vi "Text control 2 v4.3_pump-specific.vi"() -> ()   [LabVIEW 2016]
panel:
  in  "Tab Control":enum32{"Main", "Other parameters"}(tab)
  out "Line running":i32
  out "Total lines":i32
  out "Path":path=path "C:/users/rlp38/09Apr2009LTtesting/test2.txt"
  out "I vs Vg":cluster{"Y data in":dbl[], "X data in":dbl[]}[](graph)
  out "Is":dbl format="%.2e"
  out "Id":dbl format="%.2e"
  out "Ig":dbl format="%.2e"
  out "Id max vs time":cluster{"Y data in":dbl[], "X data in":dbl[]}[](graph)
  out "Id min vs time":cluster{"Y data in":dbl[], "X data in":dbl[]}[](graph)
  out "I vs Vd":cluster{"Y data in":dbl[], "X data in":dbl[]}[](graph)
  in  "Program":string="#pulsedstressV d 0.03 20 0 0.5 0.0827 5\n#\n#itime s\n#gaterangemode l\n#drainrangemode l\n#serial /1Q #query pump\n#wait 1000 #wait 1 second\n#serial /1ZR #initialize pump\n#serial /1Q #query pump\n#wait 20000 #wait 20 seconds\n#serial /1N0R #set step resolution: 0.01 mm\n#serial /1Q #query pump\n#wait 1000 #wait 1 second\n#serial /1V300R #choose speed: 300 steps/s\n#serial /1Q #query pump\n#wait 1000 #wait 1 second\n#serial /1O3R #go to port 3, counterclockwise rotation\n#serial /1Q #query pump\n#wait 1000 #wait 1 second\n#serial /1A2400R #go to absolute position 2400\n#serial /1Q #query pump\n#wait 1000 #wait 1 second\n#serial /1Q #query pump\n#serial /1? #report absolute plunger position\n#serial /1V80R #set speed to 80 steps/s\n#serial /1Q #query pump\n#serial /1O5 #switch to port 5, counterclockwise rotation\n#serial /1Q #query pump\n#wait 200 #wait 200 milliseconds\n#serial /1A0R #go to absolute position 0 (= empty syringe)\n#serial /1Q #query pump\n#serial /1? #report absolute plunger position\n#pulsed on 0.05 0 0.02\n#transfer d 1 -1 -0.1 -1 -1 0\n#wait-min 1\n#transfer d 1 -1 -0.1 -1 -1 0\n#output d 0 -1 -0.5 0 -1 -0.1\n#transfer d -10 40 1 5 40 35\n#transfer d -10 40 1 5 40 35\n#output d 0 40 20 0 40 1\n#\n#\n#sample 1 0.008 221 6 0.003\n#samplei 400e-6 200 6 0.002 0.1\n#vsu2pulse -10 4\n#\n#stressV 0.016 0.03 2e-4 0.1e-3 11\n#stressI 220e-7 0.08 15\n#transfer s -1 1 0.5 -0.005 0.005 0.005\n#output s 0 0 0 -0.008 0.008 0.002"
  out "Command running:":string="#output s 0 0 0 -0.008 0.008 0.002"
  out "Serial port data":string
  out "Elapsed Time":dbl caption="Elapsed Time (s)"
  in  "Units":u16(ring) items=["Seconds", "Minutes", "Hours"]
  in  "Time Offset":dbl caption="Set Start Time (s)"
  in  "Reset":bool
  in  "Auto Reset":bool
  in  "integration time":u32(slide) max=2 step=1 scale=0.0..2.0
  in  "Interrupt run":bool
  out "Absolute plunger position vs time":cluster{"Y data in":dbl[], "X data in":dbl[]}[](graph)
  out "Valve position vs time":cluster{"Y data in":dbl[], "X data in":dbl[]}[](graph)
  in  "Gate Range\nmode":u16(ring) items=["Auto", "Limited", "Fixed"]
  in  "Gate Range":u8(slide)=6 max=11 scale=0.0..11.0
  in  "Source/Drain\nRange mode":u16(ring) items=["Auto", "Limited", "Fixed"]
  in  "Source/Drain Range":u8(slide)=6 max=11 scale=0.0..11.0
  in  "Panel Controls":T1={"Emergency Stop"=refnum, "TransGraph Max"=1e-05, "Text/Graph (text=false)"=TRUE} {"TransGraph Max" format="%.2e"}
  in  "Panel Controls 2":T2={"Emergency Stop"=refnum, "TransGraph Max"=1e-05, "Text/Graph (text=false)"=TRUE, "TransGraph Min"=1e-11} {"TransGraph Min" format="%.2e"; "TransGraph Max" format="%.2e"}
  in  "SMU4":cluster{"on/off":bool, "Voltage":dbl} {"Voltage" min=-100.0 max=100.0 format="%.2f"}
  in  "Full Reset":bool
  in  "Standby":T3
  out "error out":errorcluster
  in  "Delay before read (ms)":u32=1000
  in  "byte count":u32=64
  in  "Serial End Mode for Reads":u16(ring)=2 items=["None", "LastBit", "TermChar"]
  in  "Timeout (ms)":u32=10000
  in  "Enable Termination\nChar (T)":bool=TRUE
  in  "Termination char\n(0xA = '\\n' = LF)\n(0xD = '\\r' = CR)":u8=13 format="%.0x"
  in  "flow control":u16(ring) items=["None"=0, "XON/XOFF"=1, "RTS/CTS"=2, "DTR/DSR"=4]
  in  "stop bits":u16(ring)=10 items=["1.0"=10, "1.5"=15, "2.0"=20]
  in  "parity":u16(ring) items=["None", "Odd", "Even", "Mark", "Space"]
  in  "data bits":u16=8 min=5 max=8 step=1
  in  "VISA resource name":refnum<visa-resource-name>="COM6"
  in  "baud rate":u32=9600
  in  "Drain: Compliance":dbl=0.001 format="%.8f"
  in  "Gate: Compliance":dbl=0.001 format="%.8f"
  in  "hold time /s":dbl format="%.2f"
  in  "delay time /s":dbl format="%.2f"
  in  "Integration time (short)":dbl=0.0019 min=8e-05 max=0.0019 step=8e-05 format="%^.0e"
  in  "Integration time (long)":dbl=0.32 min=0.04 max=2.0 step=0.02 format="%.2f"
  in  "Step delay /s":dbl format="%.2f"
  in  "Prefix (transfer)":string="_step_1_air_"
  in  "Suffix (transfer)":string="_Vg=0_T_1.txt"
  in  "Prefix (time data)":string="_buffer_Idmax_Idmin_vs_time_Vg=-1.0V_Vd=-1.0V"
  in  "Suffix (time data)":string=".txt"
  in  "Prefix (output)":string="_step_1_air_"
  in  "Suffix (output)":string="_Vg=0_O_1.txt"
  in  "Gate":T4={"Gate Start"=0.0, "Gate Stop"=2.0, "Gate Step (linear only)"=1.0, "Gate Compliance"=0.0001, "Gate PComp"=0.0, "Range mode"=0, "Range"=6} {"Range" max=11 scale=0.0..11.0; "Range mode" items=["Auto", "Limited", "Fixed"]; "Gate PComp" format="%^.2e"; "Gate Compliance" format="%^.2e"; "Gate Step (linear only)" format="%^.4e"; "Gate Stop" format="%^.4e"; "Gate Start" format="%^.4e"}
  in  "Drain 2":T5={"Drain Start"=0.0, "Drain Stop"=2.0, "Drain Compliance"=0.0001, "Drain Step"=1.0, "Drain PComp"=0.0, "Range mode"=0, "Range"=6} {"Range" max=11 scale=0.0..11.0; "Range mode" items=["Auto", "Limited", "Fixed"]; "Drain PComp" format="%^.2e"; "Drain Step" format="%^.4e"; "Drain Compliance" format="%^.2e"; "Drain Stop" format="%^.4e"; "Drain Start" format="%^.4e"}
  in  "Timings 2":T6={"integration time"=0, "Short/Long integration time"=0.00064, "hold time (sec)"=0.0, "delay time (sec)"=0.0, "Step Time (0 disables)"=0.0, "sweep method"=0, "Pulse period"=0.005, "Base voltage"=0.0, "Pulse width"=0.0005} {"Pulse width" min=0.0005 max=0.1 step=0.0001 format="%.4f"; "Base voltage" format="%^.4e"; "Pulse period" min=0.005 max=1.0 step=0.0001 format="%.4f"; "sweep method" items=["Continuous", "Pulsed"]; "Step Time (0 disables)" format="%.2f"; "delay time (sec)" format="%.4f"; "hold time (sec)" format="%.4f"; "Short/Long integration time" format="%^.0e"; "integration time" scale=0.0..2.0}
  # "Syntax:\nitime [s|m|l]\ngaterangemode [a|l|f]\ndrainrangemode [a|l|f]\npulsed [on|off] PulsePeriod(sec) PulseBaseVoltage PulseONWidth(sec)\nstandby [on l off]\nwait NumMilliseconds\nwait-min NumMinutes\n# texthere = comment\ntransfer [s|d] VgStart VgStop VgStep VdStart VdStop VdStep\noutput [s|d] VgStart VgStop VgStep VdStart VdStop VdStep\nsample Vg Vd NumSamples Time(s) SampleInterval(s)\nsamplei Idg NumSamples Time(s) SampleInterval(s) VDGcompliance\n100 samples is approximately 13 seconds with medium integration\n# if in doubt use SampleInterval(s) = 0.004\nstressV VG VD IGcompliance IDcompliance Duration(sec)\nstressI IDG VDGcompliance Duration(sec)\nvsu2pulse Bias Duration(s)\npulsedstressV [s|d] VEstop VgON VgOFF Period(s) PulseONwidth(s) Vd\nsample-fpp Vg Vd NumSamples Time\nresample-fpp Vg Vd\ntransfer-fpp [s|d] VgStart VgStop VgStep VdStart VdStop VdStep\noutput-fpp [s|d] VgStart VgStop VgStep VdStart VdStop VdStep\nserial SerialPortCommand\npump SerialPortCommand for the OEM pump\nSPM OEM Pump Syntax (<x>: pump number, use 1 if only one pump):\nif the command syntax contains [R], then append the letter R to the command\n/<x>Q: query (a query command should follow each command)\n/<x>Z[R] or /<x>Y[R]: initialize pump\n/<x>N<n>[R] (<n>=0,1): <0> (<1>) microstep 0.01 mm (0.00125 mm) resolution\n/<x>I<n> (<n>=0-6): turn to port number n (clockwise)\n/<x>O<n> (<n>=0-6): turn to port number n (counterclockwise)\n/<x>X: Re-execute last command string\n/<x>G<n>[R] (<n>=0-60000): repeat command sequence (default: 0, 0=loop forever)\n/<x>g: Mark the start of a repeat sequence (max = 10)\n/<x>M<n>[R] (<n>=0-86400000): delay command execution by n milliseconds\n/<x>H: Halt; Pause the sequence after finishing the current move\n/<x>T: Hardstop; Interrupt the current move and suppress it from the sequence\n/<x>A<n>[R] (<n>=0-3000 with N=0, 0-24000 with N=1): absolute position\n/<x>P<n>[R] (<n>=0-3000 with N=0, 0-24000 with N=1): relative pickup\n/<x>D<n>[R] (<n>=0-3000 with N=0, 0-24000 with N=1): relative dispense\n/<x>V<n>[R] (<n>=5-1600 default: 150): set peak speed (pulses/sec)\n/<x>S<n>[R] (<n>=10-40 default: 22): set speed (NOT in pulses/sec, look in manual)\nNOTE: When controlled with absolute position, one does not need to pay special attention to the syringe that is mounted on the pump.\nWithdraw from lower stage (ports 1, 3, 5), dispense from higher stage (ports 2, 4, 6)."
  # "Time"
  # "1\n2\n3\n4\n5\n6\n7\n8\n9\n10\n11\n12\n13\n14\n15\n16\n17\n18\n19\n20"
  # "Serial port settings"
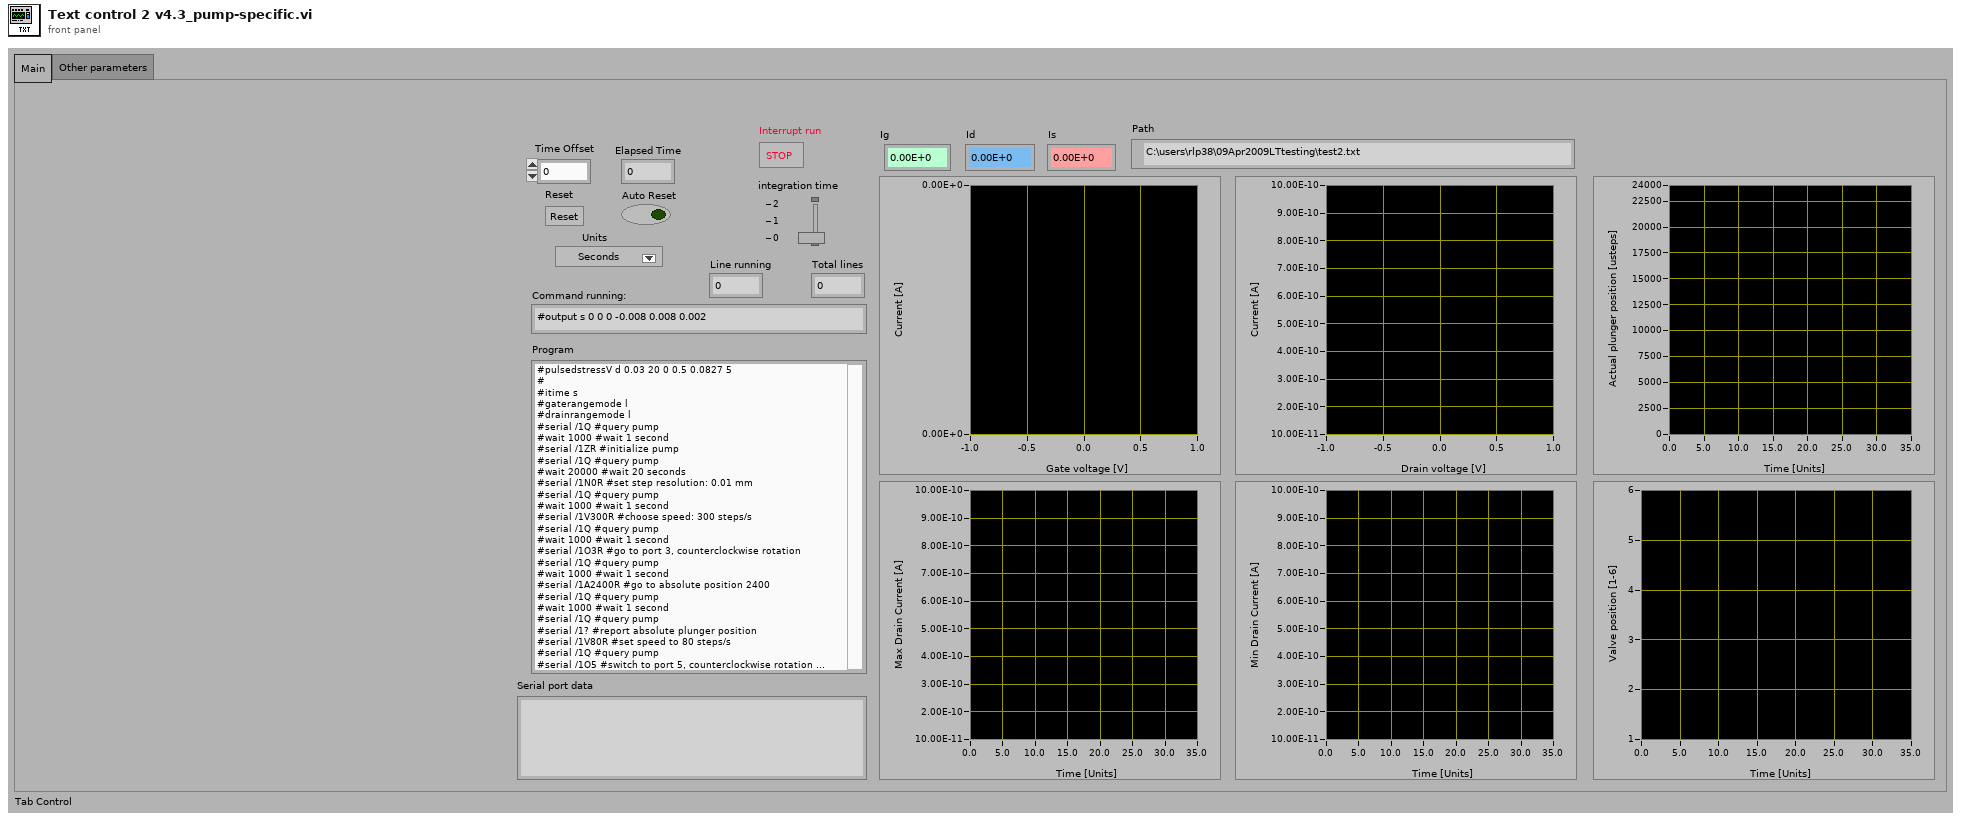
[diagram p1: front panel]
types:
  T1 = cluster{"Emergency Stop":refnum<vi>, "TransGraph Max":dbl, "Text/Graph (text=false)":bool}
  T2 = cluster{"Emergency Stop":refnum<vi>, "TransGraph Max":dbl, "Text/Graph (text=false)":bool, "TransGraph Min":dbl}
  T3 = cluster{"Gate Standby":bool, "Drain Standby":bool}
  T4 = cluster{"Gate Start":dbl, "Gate Stop":dbl, "Gate Step (linear only)":dbl, "Gate Compliance":dbl, "Gate PComp":dbl, "Range mode":u16, "Range":u8}
  T5 = cluster{"Drain Start":dbl, "Drain Stop":dbl, "Drain Compliance":dbl, "Drain Step":dbl, "Drain PComp":dbl, "Range mode":u16, "Range":u8}
  T6 = cluster{"integration time":u32, "Short/Long integration time":dbl, "hold time (sec)":dbl, "delay time (sec)":dbl, "Step Time (0 disables)":dbl, "sweep method":u16, "Pulse period":dbl, "Base voltage":dbl, "Pulse width":dbl}
  T7 = enum16{"open", "replace", "create", "open or create", "replace or create", "replace or create with confirmation"}
  T8 = cluster{"V2 Start":dbl, "V2 Step":dbl, "Number of points":i32}
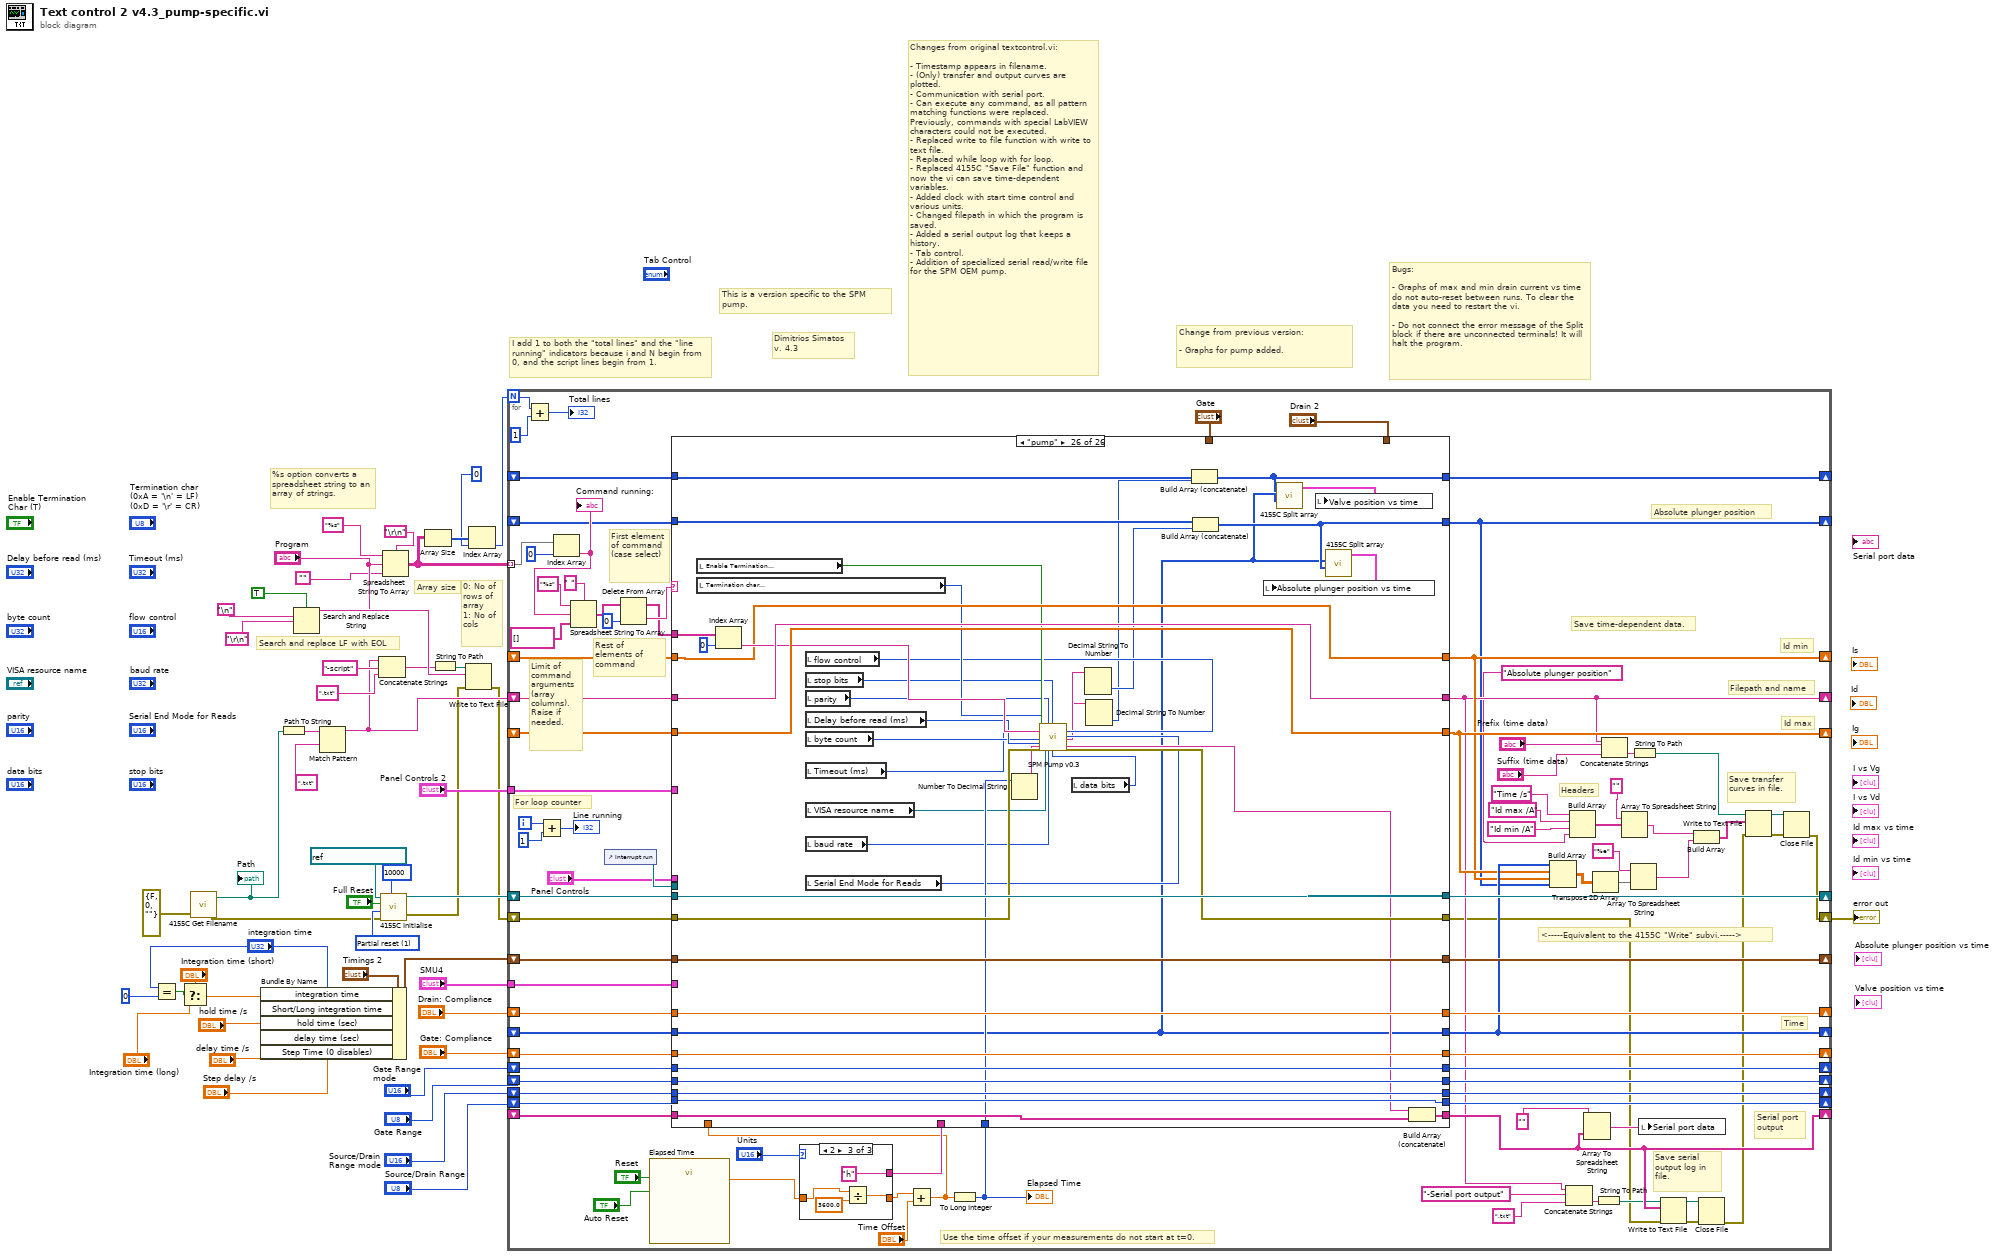
[diagram p0: block diagram]
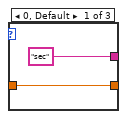
[diagram p2: hidden frame]
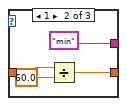
[diagram p3: hidden frame]
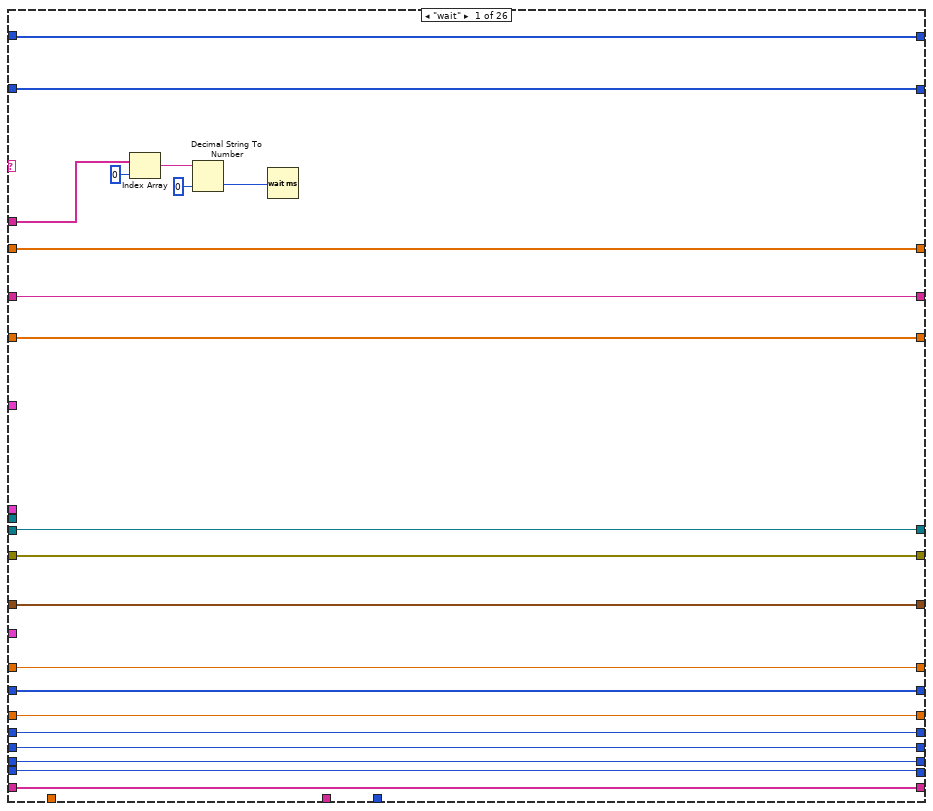
[diagram p4: hidden frame]
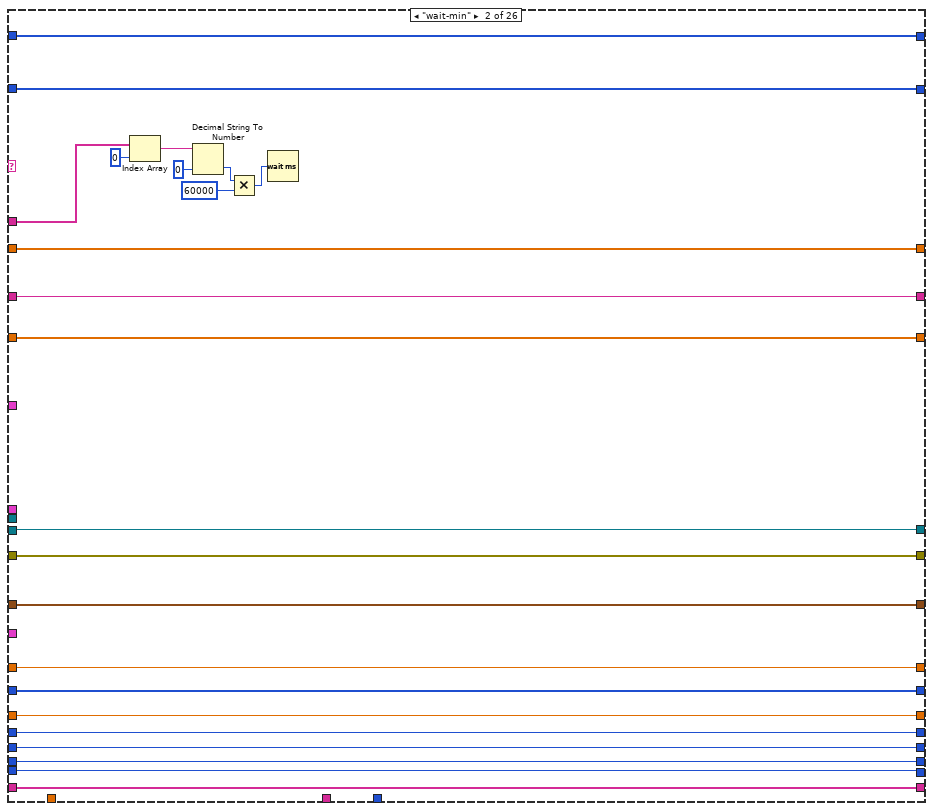
[diagram p5: hidden frame]
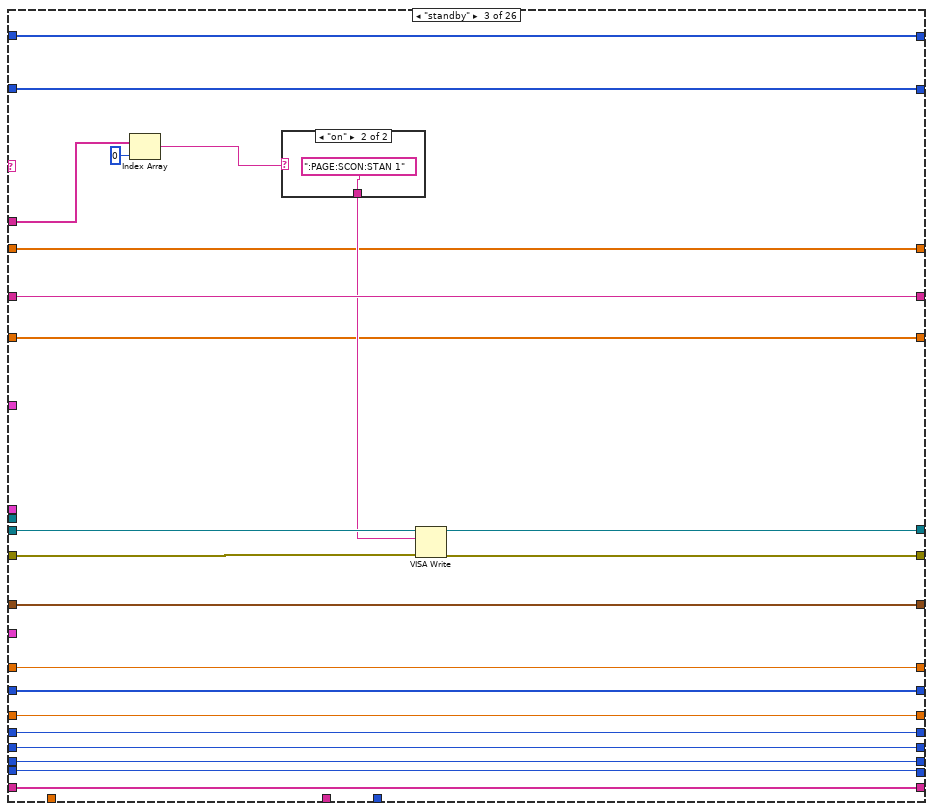
[diagram p6: hidden frame]
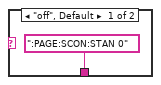
[diagram p7: hidden frame]
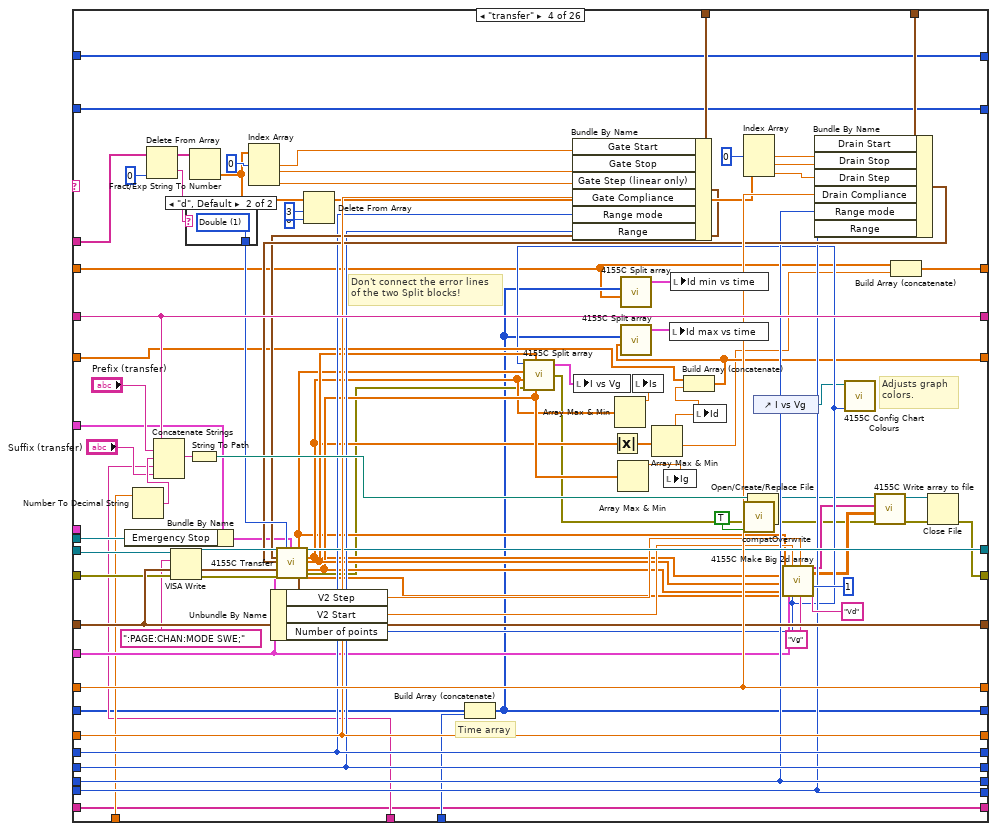
[diagram p8: hidden frame]
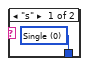
[diagram p9: hidden frame]
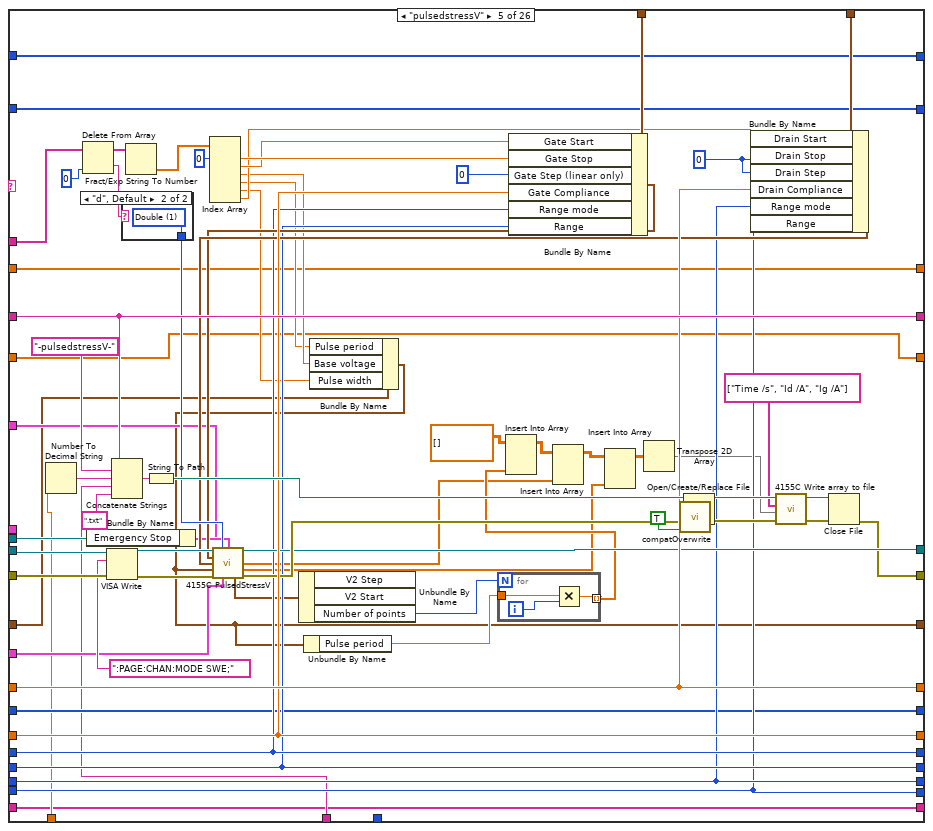
[diagram p10: hidden frame]
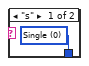
[diagram p11: hidden frame]
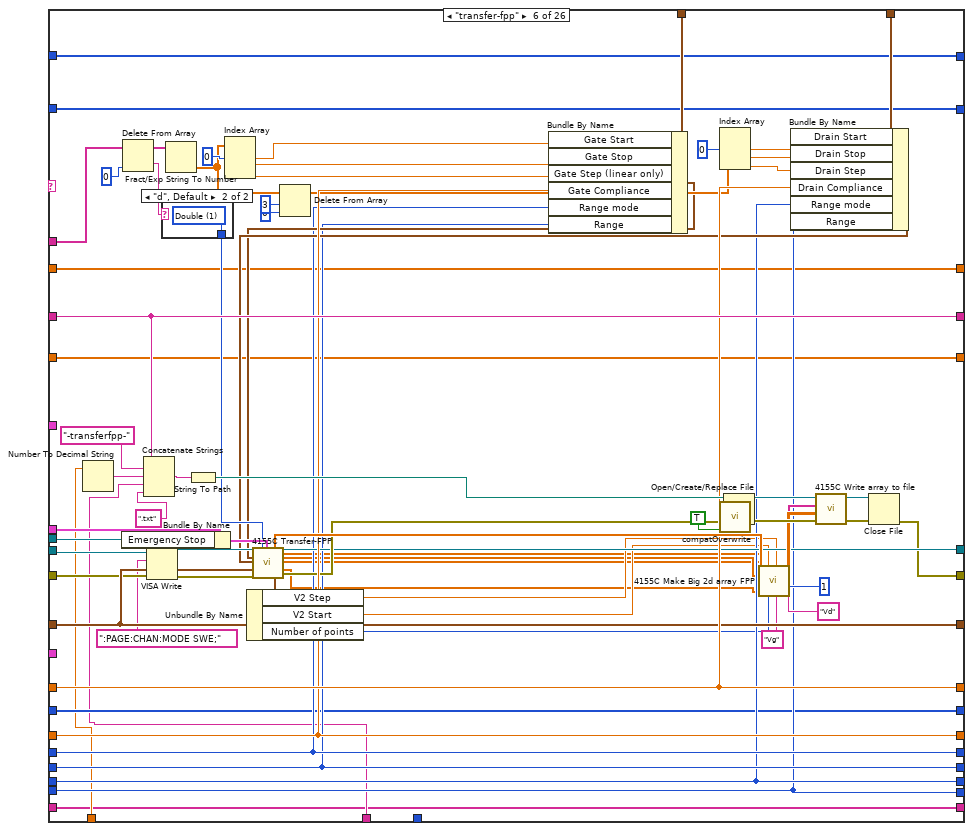
[diagram p12: hidden frame]
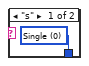
[diagram p13: hidden frame]
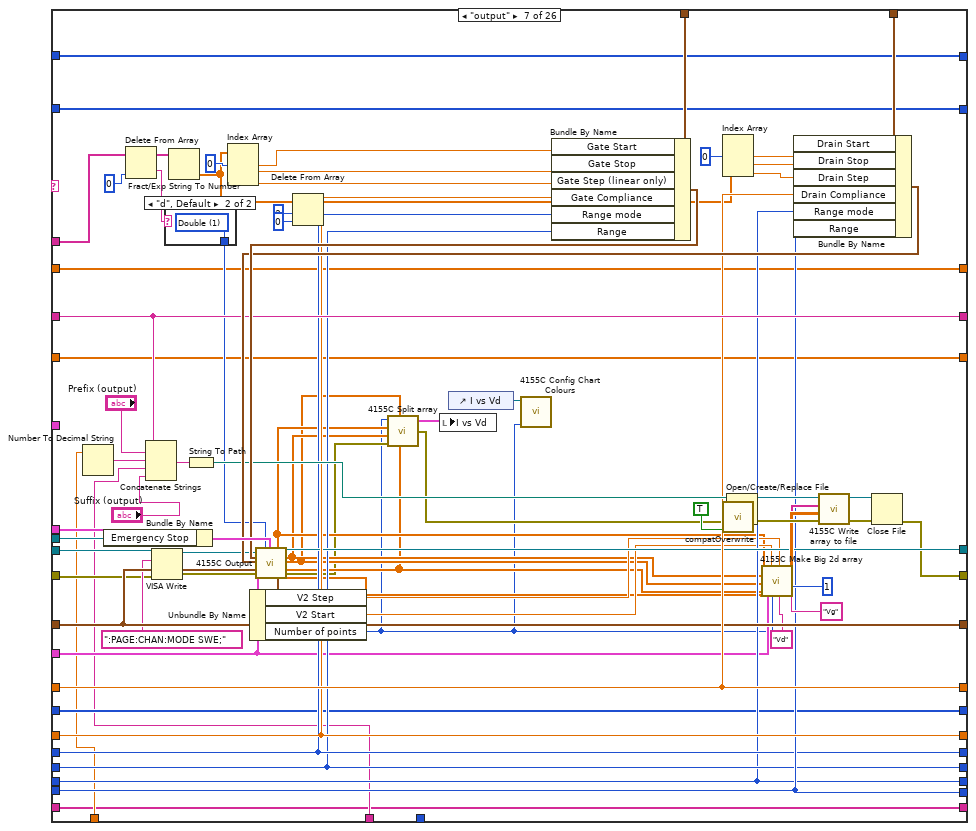
[diagram p14: hidden frame]
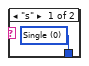
[diagram p15: hidden frame]
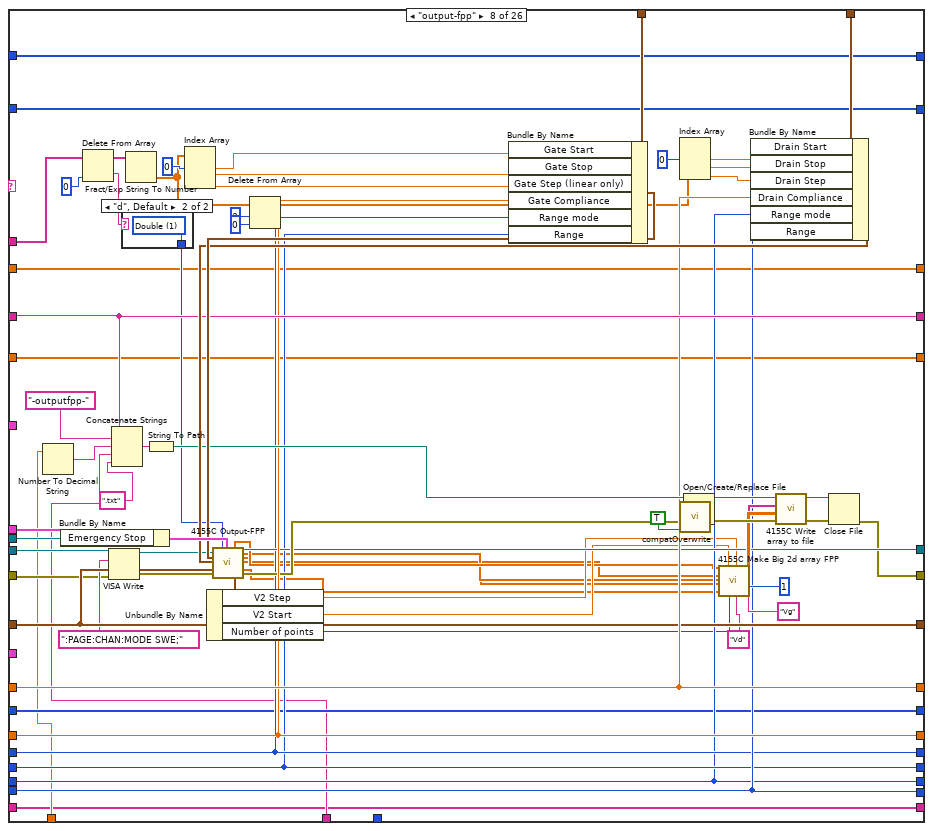
[diagram p16: hidden frame]
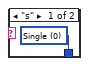
[diagram p17: hidden frame]
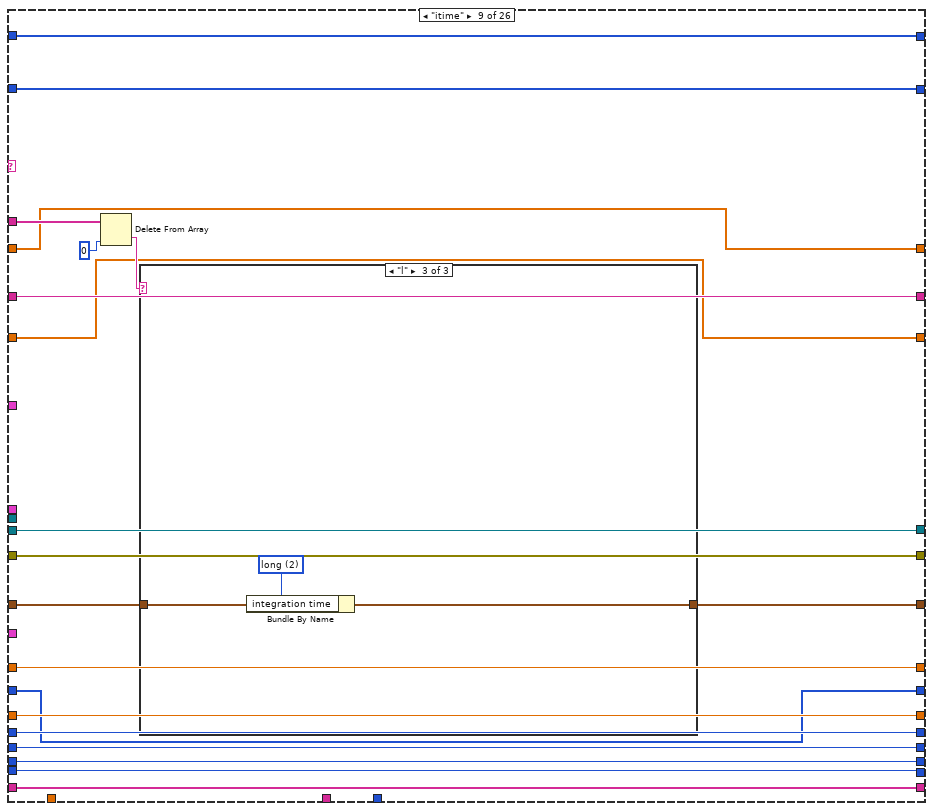
[diagram p18: hidden frame]
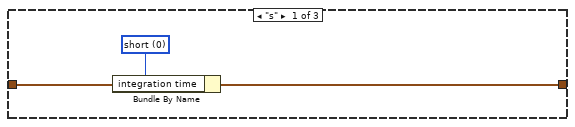
[diagram p19: hidden frame]
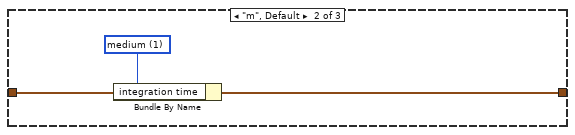
[diagram p20: hidden frame]
diagram:
  w40 = u16 1 items=["Reset All", "Partial reset"] ("Type of reset")
  # "This is a version specific to the SPM pump."
  # "I add 1 to both the \"total lines\" and the \"line running\" indicators because i and N begin from 0, and the script lines begin from 1."
  # "Bugs:\n\n- Graphs of max and min drain current vs time do not auto-reset between runs. To clear the data you need to restart the vi.\n\n- Do not connect the error message of the Split block if there are unconnected terminals! It will halt the program."
  # "Array size"
  # "%s option converts a spreadsheet string to an array of strings."
  # "0: No of rows of array\n1: No of cols"
  # "Change from previous version:\n\n- Graphs for pump added."
  # "Dimitrios Simatos\nv. 4.3"
  # "Changes from original textcontrol.vi:\n\n- Timestamp appears in filename.\n- (Only) transfer and output curves are plotted.\n- Communication with serial port.\n- Can execute any command, as all pattern matching functions were replaced. Previously, commands with special LabVIEW characters could not be executed.\n- Replaced write to file function with write to text file.\n- Replaced while loop with for loop.\n- Replaced 4155C \"Save File\" function and now the vi can save time-dependent variables.\n- Added clock with start time control and various units.\n- Changed filepath in which the program is saved.\n- Added a serial output log that keeps a history.\n- Tab control.\n- Addition of specialized serial read/write file for the SPM OEM pump."
  # "Search and replace LF with EOL"
  n1 = Equal?(x="integration time", y=u32 0) -> (x = y?=w44:bool)
  n2 = Select(t="Integration time (short)", s=w44, f="Integration time (long)") -> (s? t:f=w48:dbl)
  n3 = call "4155C Get Filename.vi"("error in (no error)"=errorcluster {"status"=FALSE, "code"=0, "source"=""}) -> ("error out"=w35:errorcluster, "path"=w10:path)  [unwired: 2 in, 1 out]
  "Path" <- w10
  n4 = Bundle By Name(cluster="Timings 2", "integration time"="integration time", "Short/Long integration time"=w48, "hold time (sec)"="hold time /s", "delay time (sec)"="delay time /s", "Step Time (0 disables)"="Step delay /s") -> (w33:T6)
  n5 = Path To String(path=w10) -> (string=w11:string)
  n6 = Search and Replace String(replace all?=TRUE ("replace all? (F)"), input string="Program", search string="\n", replace string="\r\n") -> (result string=w23:string)  [unwired: 4 in, 3 out]
  n7 = Match Pattern(string=w11, regular expression=".txt") -> (before substring=w5:string)  [unwired: 1 in, 3 out]
  n8 = Concatenate Strings(w5, "-script" ("Prefix"), ".txt" ("regular expression")) -> (w4:string)
  n9 = call "4155C Initialise.vi"("VISA resource name in"=refnum<visa-resource-name> "GPIB0::14::INSTR", "Reset"="Full Reset", "Type of reset"=w40, "error in (no error)"=w35, "VISA Timeout Value"=u32 10000) -> ("VISA Resource Name out"=w34:refnum<visa-resource-name>, "error out"=w2:errorcluster)
  n10 = Spreadsheet String To Array(delimiter (Tab)="\r\n", format string="%s", spreadsheet string="Program", array type (2D Dbl)="") -> (array=w14:string[][])
  n11 = Array Size(array=w14) -> (size(s)=w18:i32[])
  n12 = String To Path(string=w4) -> (path=w3:path)
  n13 = Write to Text File(file (use dialog)=w3, text=w23, error in=w2) -> (error out=w1:errorcluster)  [unwired: 1 in, 2 out]
  n14 = Index Array(array=w18, index=0) -> (element=w16:i32)
  n15 = for {
    N: w16 -> [w73]
    tunnel: "SMU4" -> [w118]
    shift-left: "Source/Drain Range" -> [w123]
    shift-right: [w119] -> _
    shift-left: "Source/Drain\nRange mode" -> [w124]
    shift-right: [w120] -> _
    shift-left: "Gate Range" -> [w125]
    shift-right: [w121] -> _
    shift-left: "Gate Range\nmode" -> [w126]
    shift-right: [w122] -> _
    shift-left: "Gate: Compliance" -> [w135]
    shift-right: [w131] -> _
    shift-left: "Drain: Compliance" -> [w136]
    shift-right: [w132] -> _
    shift-left: w33 -> [w137]
    shift-right: [w133] -> _
    shift-left: w1 -> [w138]
    shift-right: [w81] -> w9
    shift-left: w34 -> [w139]
    shift-right: [w134] -> _
    shift-left: w5 -> [w140]
    shift-right: [w57] -> _
    tunnel: "Panel Controls 2" -> [w117]
    shift-right: [w85] -> _
    shift-left: _ -> [w116]
    shift-right: [w86] -> _
    shift-left: _ -> [w112]
    tunnel: w14 -> [w110] mode=indexing
    shift-right: [w79] -> _
    shift-left: _ -> [w80]
    shift-right: [w62] -> _
    shift-left: _ -> [w65]
    shift-right: [w53] -> _
    shift-left: _ -> [w54]
    shift-right: [w51] -> _
    shift-left: _ -> [w50]
    i -> [w68]
    # "Absolute plunger position"
    # "Serial port output"
    # "Save serial output log in file."
    # "For loop counter"
    # "<-----Equivalent to the 4155C \"Write\" subvi.----->"
    # "Headers"
    # "Save transfer curves in file."
    # "Filepath and name"
    # "Save time-dependent data."
    # "Use the time offset if your measurements do not start at t=0."
    # "Time"
    # "Rest of elements of command"
    # "Id min"
    # "Id max"
    # "Limit of command arguments (array columns). Raise if needed."
    # "First element of command\n(case select)"
    n16 = Add(x=w73, y=1) -> (x+y=→"Total lines":i32)
    n17 = Add(x=w68, y=1) -> (x+y=→"Line running":i32)
    n18 = Index Array(array=w110, index=0 ("line index")) -> (element=w105:string)
    "Command running:" <- w105
    n19 = Spreadsheet String To Array(delimiter (Tab)=" ", format string="%s", spreadsheet string=w105, array type (2D Dbl)=string[] []) -> (array=w102:string[])
    n20 = control-ref of="Interrupt run"() -> (w130:refnum<vi>)
    n21 = Delete From Array(array=w102, index=0) -> (deleted portion=w103:string, array with subset deleted=w101:string[])  [unwired: 1 in]
    n22 = call "Elapsed Time"("Reset"="Reset", "Auto Reset"="Auto Reset") -> ("Elapsed Time (s)"=w113:dbl)  [unwired: 10 in, 7 out]
    n23 = case shown="2" "Units" {
      tunnel: ["sec" "min" "h"] -> w114
      tunnel: [w141 w145 w148] -> w75
      tunnel: w113 -> [w141 w144 w149]
      frame 0, Default {
      }
      frame 1 {
        n24 = Divide(x=w144, y=60.0) -> (x/y=w145:dbl)
      }
      frame 2 {
        n25 = Divide(x=w149, y=3600.0) -> (x/y=w148:dbl)
      }
    }
    n26 = Add(x=w75, y="Time Offset") -> (x+y=w74:dbl)
    n27 = To Long Integer(number=w74) -> (32bit integer=w111:i32)
    "Elapsed Time" <- w111
    n28 = case shown="\"pump\"" w103 {
      tunnel: w101 -> [w171 w194 w216 w295 w363 w436 w515 w589 w631 w661 w692 w721 w746 w764 _ _ w880 w945 _ w1018 w1066 w1112 w1186 w1252 w1276 w1321]
      tunnel: w140 -> [w166 w190 w214 w302 w370 w444 w522 w597 w620 w650 w684 w714 w740 w757 w780 w826 w858 w927 w962 w1005 w1053 w1100 w1180 w1248 w1278 w1323]
      tunnel: w139 -> [w165 w189 w205 w273 w354 w413 w491 w565 w621 w651 w685 w715 w741 w758 w785 w828 w886 w951 w966 w1024 w1072 w1118 w1192 w1206 w1282 w1327]
      tunnel: w138 -> [w164 w188 w204 w272 w353 w412 w488 w562 w622 w652 w686 w716 w742 w759 w784 w799 w885 w950 w965 w1023 w1071 w1117 w1191 w1205 w1281 w1326]
      tunnel: w137 -> [w163 w187 w213 w298 w329 w440 w518 w593 w630 w660 w683 w713 w739 w756 w783 w823 w849 w919 w971 w998 w1046 w1093 w1179 w1247 w1283 w1328]
      tunnel: w136 -> [w162 w186 w212 w300 w368 w442 w520 w595 w629 w659 w691 w720 w745 w763 w782 w808 w884 w949 w974 w1022 w1070 w1116 w1190 w1256 w1284 w1329]
      tunnel: w135 -> [w161 w185 w211 w299 w367 w441 w519 w594 w628 w658 w690 w719 w744 w762 w781 w809 w859 w928 w973 w1006 w1054 w1101 w1181 w1249 w1286 w1330]
      tunnel: [w165 w189 w203 w297 w365 w438 w517 w591 w621 w651 w685 w715 w741 w758 w785 w828 w850 w901 w964 w999 w1047 w1094 w1132 w1208 w1282 w1327] -> w134
      tunnel: [w164 w188 w202 w296 w364 w437 w516 w590 w622 w652 w686 w716 w742 w759 w784 w798 w860 w902 w963 w1007 w1055 w1102 w1131 w1207 w1280 w1325] -> w56
      tunnel: [w163 w187 w213 w298 w325 w440 w518 w593 w623 w653 w683 w713 w739 w756 w783 w823 w849 w919 w971 w998 w1046 w1093 w1179 w1247 w1283 w1328] -> w133
      tunnel: [w162 w186 w212 w300 w368 w442 w520 w595 w629 w659 w691 w720 w745 w763 w782 w808 w884 w949 w974 w1022 w1070 w1116 w1190 w1256 w1284 w1329] -> w132
      tunnel: [w161 w185 w211 w299 w367 w441 w519 w594 w628 w658 w690 w719 w744 w762 w781 w809 w859 w928 w973 w1006 w1054 w1101 w1181 w1249 w1286 w1330] -> w131
      tunnel: [w166 w190 w214 w302 w370 w444 w522 w597 w620 w650 w684 w714 w740 w757 w780 w826 w858 w927 w962 w1005 w1053 w1100 w1180 w1248 w1278 w1323] -> w57
      tunnel: w130 -> [_ _ _ w305 w374 w449 w526 w601 _ _ _ _ _ _ _ _ w855 w924 _ w1004 w1052 w1099 w1152 w1224 _ _]
      tunnel: "Gate" -> [_ _ _ w282 w357 w423 w502 w576 _ _ _ _ _ _ _ _ _ _ _ _ _ _ _ _ _ _]
      tunnel: "Drain 2" -> [_ _ _ w281 w356 w422 w501 w575 _ _ _ _ _ _ _ _ _ _ _ _ _ _ _ _ _ _]
      tunnel: "Panel Controls" -> [_ _ _ _ _ w421 w500 w574 _ _ _ _ _ _ _ _ _ _ _ _ _ _ _ _ _ _]
      tunnel: w126 -> [w160 w184 w210 w266 w347 w406 w486 w560 w627 w657 _ w712 w738 w755 w779 w810 w845 w915 w967 w994 w1042 w1089 w1175 w1243 w1287 w1331]
      tunnel: w125 -> [w159 w183 w209 w265 w346 w405 w485 w559 w626 w656 w689 _ w729 w761 w778 w811 w846 w916 w968 w995 w1043 w1090 w1176 w1244 w1288 w1332]
      tunnel: w124 -> [w158 w182 w208 w264 w345 w404 w484 w558 w625 w655 w688 w718 w743 _ w777 w812 w847 w917 w969 w996 w1044 w1091 w1177 w1245 w1289 w1333]
      tunnel: w123 -> [w157 w181 w207 w263 w344 w403 w487 w561 w624 w654 w687 w717 _ w760 w776 w813 w848 w918 w970 w997 w1045 w1092 w1178 w1246 w1290 w1334]
      tunnel: [w160 w184 w210 w266 w347 w406 w486 w560 w627 w657 w682 w712 w738 w755 w779 w810 w845 w915 w967 w994 w1042 w1089 w1175 w1243 w1287 w1331] -> w122
      tunnel: [w159 w183 w209 w265 w346 w405 w485 w559 w626 w656 w689 w704 w729 w761 w778 w811 w846 w916 w968 w995 w1043 w1090 w1176 w1244 w1288 w1332] -> w121
      tunnel: [w158 w182 w208 w264 w345 w404 w484 w558 w625 w655 w688 w718 w743 w754 w777 w812 w847 w917 w969 w996 w1044 w1091 w1177 w1245 w1289 w1333] -> w120
      tunnel: [w157 w181 w207 w263 w344 w403 w487 w561 w624 w654 w687 w717 w730 w760 w776 w813 w848 w918 w970 w997 w1045 w1092 w1178 w1246 w1290 w1334] -> w119
      tunnel: w118 -> [_ _ _ w258 w341 _ w480 _ _ _ _ _ _ _ _ _ _ _ _ _ _ _ _ _ _ _]
      tunnel: w117 -> [_ _ _ w256 w340 _ _ _ _ _ _ _ _ _ _ _ _ _ _ _ _ _ _ _ _ _]
      tunnel: [w156 w177 w200 w233 w317 w393 w477 w547 w619 w648 w681 w703 w728 w753 w775 w794 w837 w899 w961 w983 w1035 w1083 w1129 w1201 w1279 w1324] -> w85
      tunnel: w116 -> [w156 w177 w200 w247 w317 w393 w477 w547 w619 w648 w681 w703 w728 w753 w775 w794 w837 w899 w961 w983 w1035 w1083 w1129 w1201 w1279 w1324]
      tunnel: w74 -> [_ _ _ w243 w314 w391 w474 w544 _ _ _ _ _ _ _ w792 w835 w896 _ w980 w1032 w1080 w1126 w1197 _ _]
      tunnel: w114 -> [_ _ _ w240 w313 w389 w473 w543 _ _ _ _ _ _ _ w790 w833 w895 _ w979 w1031 w1079 w1125 w1198 _ _]
      tunnel: w111 -> [_ _ _ w234 _ _ _ _ _ _ _ _ _ _ _ _ _ _ _ _ _ _ _ _ _ w1316]
      tunnel: [w155 w176 w199 w231 w316 w392 w476 w546 w618 w647 w680 w702 w727 w752 w774 w793 w836 w898 w960 w982 w1034 w1082 w1128 w1200 w1285 w1296] -> w86
      tunnel: w112 -> [w155 w176 w199 w239 w316 w392 w476 w546 w618 w647 w680 w702 w727 w752 w774 w793 w836 w898 w960 w982 w1034 w1082 w1128 w1200 w1285 w1296]
      tunnel: [w154 w175 w198 w229 w312 w388 w472 w542 w617 w646 w679 w701 w726 w751 w773 w789 w832 w894 w959 w978 w1030 w1078 w1124 w1196 w1274 w1319] -> w79
      tunnel: w80 -> [w154 w175 w198 w228 w312 w388 w472 w542 w617 w646 w679 w701 w726 w751 w773 w789 w832 w894 w959 w978 w1030 w1078 w1124 w1196 w1274 w1319]
      tunnel: [w153 w174 w197 w221 w311 w387 w462 w541 w616 w645 w678 w700 w725 w750 w772 w788 w831 w893 w958 w977 w1029 w1077 w1123 w1195 w1273 w1318] -> w62
      tunnel: w65 -> [w153 w174 w197 w221 w311 w387 w462 w541 w616 w645 w678 w700 w725 w750 w772 w788 w831 w893 w958 w977 w1029 w1077 w1123 w1195 w1272 w1317]
      tunnel: [w152 w173 w196 w220 w310 w386 w461 w540 w615 w644 w677 w699 w724 w749 w771 w787 w830 w892 w957 w976 w1028 w1076 w1122 w1194 w1258 w1298] -> w53
      tunnel: w54 -> [w152 w173 w196 w220 w310 w386 w461 w540 w615 w644 w677 w699 w724 w749 w771 w787 w830 w892 w957 w976 w1028 w1076 w1122 w1194 w1258 w1297]
      tunnel: [w151 w172 w195 w219 w309 w385 w460 w539 w614 w643 w676 w698 w723 w748 w770 w786 w829 w891 w956 w975 w1027 w1075 w1121 w1193 w1257 w1292] -> w51
      tunnel: w50 -> [w151 w172 w195 w219 w309 w385 w460 w539 w614 w643 w676 w698 w723 w748 w770 w786 w829 w891 w956 w975 w1027 w1075 w1121 w1193 w1257 w1291]
      frame "wait" {
        n29 = Index Array(array=w171, index=0 ("Index")) -> (element=w169:string)
        n30 = Decimal String To Number(string=w169, default (0L)=u32 0) -> (number=w168:u32)  [unwired: 1 in, 1 out]
        n31 = Wait (ms)(milliseconds to wait=w168) -> ()  [unwired: 1 out]
      }
      frame "wait-min" {
        n32 = Index Array(array=w194, index=0 ("Index")) -> (element=w192:string)
        n33 = Decimal String To Number(string=w192, default (0L)=u32 0) -> (number=w180:u32)  [unwired: 1 in, 1 out]
        n34 = Multiply(x=w180, y=u32 60000) -> (x*y=w179:u32)
        n35 = Wait (ms)(milliseconds to wait=w179) -> ()  [unwired: 1 out]
      }
      frame "standby" {
        n36 = Index Array(array=w216, index=0 ("Index")) -> (element=w206:string)
        n37 = case shown="\"on\"" w206 {
          tunnel: [":PAGE:SCON:STAN 0" ":PAGE:SCON:STAN 1"] -> w201
          frame "off", Default {
          }
          frame "on" {
          }
        }
        n38 = VISA Write(VISA resource name=w205, write buffer=w201, error in (no error)=w204) -> (VISA resource name out=w203:refnum<visa-resource-name>, error out=w202:errorcluster)  [unwired: 1 out]
      }
      frame "transfer" {
        # "Don't connect the error lines\nof the two Split blocks!"
        # "Adjusts graph colors."
        # "Time array"
        n39 = Bundle By Name(cluster=w256, "Emergency Stop"=w305) -> (w257:T2)
        n40 = Number To Decimal String(number=w243) -> (decimal integer string=w242:string)  [unwired: 1 in]
        n41 = Delete From Array(array=w295, index=0 ("Index")) -> (deleted portion=w293:string, array with subset deleted=w292:string[])  [unwired: 1 in]
        n42 = Concatenate Strings(w302, "Prefix (transfer)", w242, w240, "Suffix (transfer)") -> (w304:string)
        n43 = VISA Write(VISA resource name=w273, write buffer=":PAGE:CHAN:MODE SWE;" ("write buffer (\"\")"), error in (no error)=w272) -> (VISA resource name out=w270:refnum<visa-resource-name>, error out=w271:errorcluster)  [unwired: 1 out]
        n44 = case shown="\"d\", Default" w293 {
          tunnel: [w307 w308] -> w291
          frame "s" {
            w307 = u16 0 items=["Single", "Double"] ("sweep mode")
          }
          frame "d", Default {
            w308 = u16 1 items=["Single", "Double"] ("sweep mode")
          }
        }
        n45 = String To Path(string=w304) -> (path=w301:path)
        n46 = Fract/Exp String To Number(string=w292) -> (number=w277:dbl[])  [unwired: 3 in, 1 out]
        n47 = Index Array(array=w277, index #1=0 ("Index")) -> (element #1=w290:dbl, element #2=w289:dbl, element #3=w288:dbl)  [unwired: 2 in]
        n48 = Delete From Array(array=w277, length=3 ("Length"), index=0 ("Index")) -> (array with subset deleted=w275:dbl[])  [unwired: 1 out]
        n49 = Build Array (concatenate)(w239, w234) -> (w231:i32[])
        n50 = Bundle By Name(cluster=w282, "Gate Start"=w290, "Gate Stop"=w289, "Gate Step (linear only)"=w288, "Gate Compliance"=w299, "Range mode"=w266, "Range"=w265) -> (w267:T4)
        n51 = call "4155C Split array.vi"("X data in"=w231, "Y1 data in"=w228) -> ("Array of clusters"=w232:cluster{"Y data in":dbl[], "X data in":dbl[]}[])  [unwired: 5 in, 1 out]
        n52 = local write "Id min vs time"(w232) -> ()
        n53 = Index Array(array=w275, index #1=0 ("Index")) -> (element #1=w285:dbl, element #2=w284:dbl, element #3=w283:dbl)  [unwired: 2 in]
        n54 = call <vilib>:"compatOverwrite.vi"("overwrite (F)"=TRUE) -> ("overwrite?"=w255:T7)
        n55 = control-ref of="I vs Vg"() -> (w244:refnum<vi>)
        n56 = Bundle By Name(cluster=w281, "Drain Start"=w285, "Drain Stop"=w284, "Drain Step"=w283, "Drain Compliance"=w300, "Range mode"=w264, "Range"=w263) -> (w268:T5)
        n57 = call "4155C Transfer.vi"("VISA resource name in"=w270, "Gate"=w267, "Drain"=w268, "Timings"=w298, "error in (no error)"=w271, "SMU4"=w258, "sweep mode"=w291, "Panel Controls"=w257) -> ("VG"=w248:dbl[], "Outparams"=w262:T8, "VISA Resource Name out"=w297:refnum<visa-resource-name>, "IS"=w249:dbl[], "ID"=w254:dbl[], "IG"=w250:dbl[], "error out"=w235:errorcluster, "SMU4"=w259:dbl[])  [unwired: 12 in]
        n58 = Unbundle By Name(w262) -> ("V2 Step"=w261:dbl, "V2 Start"=w260:dbl, "Number of points"=w245:i32)
        n59 = call "4155C Split array.vi"("Number of VAR2 steps"=w245, "Y2 data in"=w254, "X data in"=w248, "Y1 data in"=w249, "Y3 data in"=w250, "error in (no error)"=w235) -> ("Array of clusters"=w238:cluster{"Y data in":dbl[], "X data in":dbl[]}[], "error out"=w236:errorcluster)  [unwired: 1 in]
        n60 = local write "I vs Vg"(w238) -> ()
        n61 = Absolute Value(x=w249) -> (abs(x)=w253:dbl[])
        n62 = Array Max & Min(array=w249) -> (max value=w251:dbl)  [unwired: 3 out]
        n63 = Array Max & Min(array=w250) -> (max value=w252:dbl)  [unwired: 3 out]
        n64 = local write "Is"(w251) -> ()
        n65 = Array Max & Min(array=w253) -> (max value=w246:dbl, min value=w230:dbl)  [unwired: 2 out]
        n66 = local write "Ig"(w252) -> ()
        n67 = Build Array (concatenate)(w247, w246) -> (w233:dbl[])
        n68 = call "4155C Split array.vi"("X data in"=w231, "Y1 data in"=w233) -> ("Array of clusters"=w237:cluster{"Y data in":dbl[], "X data in":dbl[]}[])  [unwired: 5 in, 1 out]
        n69 = local write "Id max vs time"(w237) -> ()
        n70 = local write "Id"(w246) -> ()
        n71 = Open/Create/Replace File(file path (use dialog)=w301, error in=w236, operation (0:open)=w255) -> (refnum out=w226:refnum<file>, error out=w224:errorcluster)  [unwired: 3 in, 1 out]
        n72 = call "4155C Make Big 2d array.vi"("1D Var1"=w248, "1d IS"=w249, "1d ID"=w254, "1d IG"=w250, "1d SMU4"=w259, "SMU4"=w258, "VAR2 START"=w260, "Number of VAR2 steps"=w245, "VAR2 STEP"=w261, "VAR1 Name"="Vg", "Decimal places in header"=i8 1, "VAR2 Name"="Vd") -> ("Header array"=w227:string[], "Data array"=w225:dbl[][])  [unwired: 14 in]
        n73 = call "4155C Config Chart Colours.vi"("Numeric"=w245, "XY Graph 2"=w244) -> ()  [unwired: 6 in]
        n74 = call "4155C Write array to file.vi"("Byte Stream File Refnum"=w226, "Header"=w227, "Data Array"=w225, "error in (no error)"=w224) -> ("dup refnum"=w223:refnum<file>, "error out"=w222:errorcluster)  [unwired: 1 in]
        n75 = Build Array (concatenate)(w228, w230) -> (w229:dbl[])
        n76 = Close File(refnum=w223, error in=w222) -> (error out=w296:errorcluster)  [unwired: 1 out]
      }
      frame "pulsedstressV" {
        w323 = 0
        n77 = Number To Decimal String(number=w314) -> (decimal integer string=w371:string)  [unwired: 1 in]
        n78 = Delete From Array(array=w363, index=0 ("Index")) -> (deleted portion=w361:string, array with subset deleted=w360:string[])  [unwired: 1 in]
        n79 = Bundle By Name(cluster=w340, "Emergency Stop"=w374) -> (w342:T2)
        n80 = VISA Write(VISA resource name=w354, write buffer=":PAGE:CHAN:MODE SWE;" ("write buffer (\"\")"), error in (no error)=w353) -> (VISA resource name out=w351:refnum<visa-resource-name>, error out=w352:errorcluster)  [unwired: 1 out]
        n81 = Concatenate Strings(w370, "-pulsedstressV-" ("Substring"), w371, w313, ".txt" ("Substring")) -> (w373:string)
        n82 = case shown="\"d\", Default" w361 {
          tunnel: [w383 w384] -> w359
          frame "s" {
            w383 = u16 0 items=["Single", "Double"] ("sweep mode")
          }
          frame "d", Default {
            w384 = u16 1 items=["Single", "Double"] ("sweep mode")
          }
        }
        n83 = Fract/Exp String To Number(string=w360) -> (number=w355:dbl[])  [unwired: 3 in, 1 out]
        n84 = String To Path(string=w373) -> (path=w369:path)
        n85 = Index Array(array=w355, index #1=0 ("Index")) -> (element #1=w332:dbl, element #2=w331:dbl, element #3=w328:dbl, element #4=w327:dbl, element #5=w326:dbl, element #6=w330:dbl)  [unwired: 5 in]
        n86 = Bundle By Name(cluster=w329, "Pulse period"=w327, "Base voltage"=w328, "Pulse width"=w326) -> (w325:T6)
        n87 = Unbundle By Name(w325) -> ("Pulse period"=w333:dbl)
        n88 = Bundle By Name(cluster=w357, "Gate Start"=w331, "Gate Stop"=w332, "Gate Step (linear only)"=0, "Gate Compliance"=w367, "Range mode"=w347, "Range"=w346) -> (w348:T4)
        n89 = call <vilib>:"compatOverwrite.vi"("overwrite (F)"=TRUE) -> ("overwrite?"=w318:T7)
        n90 = Bundle By Name(cluster=w356, "Drain Start"=w330, "Drain Stop"=w323, "Drain Step"=w323, "Drain Compliance"=w368, "Range mode"=w345, "Range"=w344) -> (w349:T5)
        n91 = call "4155C PulsedStressV.vi"("VISA resource name in"=w351, "sweep mode"=w359, "Panel Controls"=w342, "Gate"=w348, "Drain"=w349, "Timings"=w325, "error in (no error)"=w352, "SMU4"=w341) -> ("VISA Resource Name out"=w365:refnum<visa-resource-name>, "ID"=w321:dbl[], "IG"=w319:dbl[], "Outparams"=w343:T8, "error out"=w366:errorcluster)  [unwired: 3 in]
        n92 = Unbundle By Name(w343) -> ("Number of points"=w320:i32)  [unwired: 2 out]
        n93 = for {
          N: w320 -> [_]
          tunnel: [w380] -> w322 mode=indexing
          tunnel: w333 -> [w382]
          i -> [w381]
          n94 = Multiply(x=w382, y=w381) -> (x*y=w380:dbl)
        }
        n95 = Insert Into Array(array=dbl[][] [] ("Input Array"), new element=w322) -> (w334:dbl[][])  [unwired: 2 in]
        n96 = Insert Into Array(array=w334, new element=w321) -> (w339:dbl[][])  [unwired: 2 in]
        n97 = Insert Into Array(array=w339, new element=w319) -> (w338:dbl[][])  [unwired: 2 in]
        n98 = Transpose 2D Array(2D array=w338) -> (transposed array=w337:dbl[][])
        n99 = Open/Create/Replace File(file path (use dialog)=w369, error in=w366, operation (0:open)=w318) -> (refnum out=w377:refnum<file>, error out=w378:errorcluster)  [unwired: 3 in, 1 out]
        n100 = call "4155C Write array to file.vi"("Byte Stream File Refnum"=w377, "Header"=string[] ["Time /s", "Id /A", "Ig /A"], "Data Array"=w337, "error in (no error)"=w378) -> ("dup refnum"=w375:refnum<file>, "error out"=w376:errorcluster)  [unwired: 1 in]
        n101 = Close File(refnum=w375, error in=w376) -> (error out=w364:errorcluster)  [unwired: 1 out]
      }
      frame "transfer-fpp" {
        n102 = Number To Decimal String(number=w391) -> (decimal integer string=w445:string)  [unwired: 1 in]
        n103 = Bundle By Name(cluster=w421, "Emergency Stop"=w449) -> (w457:T1)
        n104 = Delete From Array(array=w436, index=0 ("Index")) -> (deleted portion=w434:string, array with subset deleted=w433:string[])  [unwired: 1 in]
        n105 = Concatenate Strings(w444, "-transferfpp-" ("Substring"), w445, w389, ".txt" ("Substring")) -> (w447:string)
        n106 = VISA Write(VISA resource name=w413, write buffer=":PAGE:CHAN:MODE SWE;" ("write buffer (\"\")"), error in (no error)=w412) -> (VISA resource name out=w410:refnum<visa-resource-name>, error out=w411:errorcluster)  [unwired: 1 out]
        n107 = case shown="\"d\", Default" w434 {
          tunnel: [w458 w459] -> w432
          frame "s" {
            w458 = u16 0 items=["Single", "Double"] ("sweep mode")
          }
          frame "d", Default {
            w459 = u16 1 items=["Single", "Double"] ("sweep mode")
          }
        }
        n108 = Fract/Exp String To Number(string=w433) -> (number=w417:dbl[])  [unwired: 3 in, 1 out]
        n109 = String To Path(string=w447) -> (path=w443:path)
        n110 = Index Array(array=w417, index #1=0 ("Index")) -> (element #1=w431:dbl, element #2=w430:dbl, element #3=w429:dbl)  [unwired: 2 in]
        n111 = Delete From Array(array=w417, length=3 ("Length"), index=0 ("Index")) -> (array with subset deleted=w415:dbl[])  [unwired: 1 out]
        n112 = Bundle By Name(cluster=w423, "Gate Start"=w431, "Gate Stop"=w430, "Gate Step (linear only)"=w429, "Gate Compliance"=w441, "Range mode"=w406, "Range"=w405) -> (w407:T4)
        n113 = Index Array(array=w415, index #1=0 ("Index")) -> (element #1=w426:dbl, element #2=w425:dbl, element #3=w424:dbl)  [unwired: 2 in]
        n114 = call <vilib>:"compatOverwrite.vi"("overwrite (F)"=TRUE) -> ("overwrite?"=w394:T7)
        n115 = Bundle By Name(cluster=w422, "Drain Start"=w426, "Drain Stop"=w425, "Drain Step"=w424, "Drain Compliance"=w442, "Range mode"=w404, "Range"=w403) -> (w408:T5)
        n116 = call "4155C Transfer-FPP.vi"("VISA resource name in"=w410, "Gate"=w407, "Drain"=w408, "Timings"=w440, "error in (no error)"=w411, "sweep mode"=w432, "Panel Controls"=w457) -> ("VG"=w448:dbl[], "Outparams"=w402:T8, "VISA Resource Name out"=w438:refnum<visa-resource-name>, "Vprobe2"=w398:dbl[], "ID"=w397:dbl[], "IG"=w396:dbl[], "Vprobe1"=w395:dbl[], "error out"=w439:errorcluster)  [unwired: 13 in]
        n117 = Unbundle By Name(w402) -> ("V2 Step"=w401:dbl, "V2 Start"=w400:dbl, "Number of points"=w399:i32)
        n118 = Open/Create/Replace File(file path (use dialog)=w443, error in=w439, operation (0:open)=w394) -> (refnum out=w454:refnum<file>, error out=w455:errorcluster)  [unwired: 3 in, 1 out]
        n119 = call "4155C Make Big 2d array FPP.vi"("1D Var1"=w448, "1d ID"=w397, "1d Vp2"=w398, "1d IG"=w396, "1d Vp1"=w395, "VAR2 START"=w400, "Number of VAR2 steps"=w399, "VAR2 STEP"=w401, "VAR1 Name"="Vg", "Decimal places in header"=i8 1, "VAR2 Name"="Vd") -> ("Header array"=w450:string[], "Data array"=w451:dbl[][])  [unwired: 15 in]
        n120 = call "4155C Write array to file.vi"("Byte Stream File Refnum"=w454, "Header"=w450, "Data Array"=w451, "error in (no error)"=w455) -> ("dup refnum"=w452:refnum<file>, "error out"=w453:errorcluster)  [unwired: 1 in]
        n121 = Close File(refnum=w452, error in=w453) -> (error out=w437:errorcluster)  [unwired: 1 out]
      }
      frame "output" {
        n122 = Number To Decimal String(number=w474) -> (decimal integer string=w523:string)  [unwired: 1 in]
        n123 = Bundle By Name(cluster=w500, "Emergency Stop"=w526) -> (w536:T1)
        n124 = Delete From Array(array=w515, index=0 ("Index")) -> (deleted portion=w513:string, array with subset deleted=w512:string[])  [unwired: 1 in]
        n125 = Concatenate Strings(w522, "Prefix (output)", w523, w473, "Suffix (output)") -> (w525:string)
        n126 = VISA Write(VISA resource name=w491, write buffer=":PAGE:CHAN:MODE SWE;" ("write buffer (\"\")"), error in (no error)=w488) -> (VISA resource name out=w490:refnum<visa-resource-name>, error out=w489:errorcluster)  [unwired: 1 out]
        n127 = case shown="\"d\", Default" w513 {
          tunnel: [w537 w538] -> w511
          frame "s" {
            w537 = u16 0 items=["Single", "Double"] ("sweep mode")
          }
          frame "d", Default {
            w538 = u16 1 items=["Single", "Double"] ("sweep mode")
          }
        }
        n128 = Fract/Exp String To Number(string=w512) -> (number=w494:dbl[])  [unwired: 3 in, 1 out]
        n129 = String To Path(string=w525) -> (path=w521:path)
        n130 = Index Array(array=w494, index #1=0 ("Index")) -> (element #1=w510:dbl, element #2=w509:dbl, element #3=w508:dbl)  [unwired: 2 in]
        n131 = Delete From Array(array=w494, length=3 ("Length"), index=0 ("Index")) -> (array with subset deleted=w493:dbl[])  [unwired: 1 out]
        n132 = control-ref of="I vs Vd"() -> (w464:refnum<vi>)
        n133 = Bundle By Name(cluster=w502, "Gate Start"=w510, "Gate Stop"=w509, "Gate Step (linear only)"=w508, "Gate Compliance"=w519, "Range mode"=w486, "Range"=w485) -> (w535:T4)
        n134 = Index Array(array=w493, index #1=0 ("Index")) -> (element #1=w505:dbl, element #2=w504:dbl, element #3=w503:dbl)  [unwired: 2 in]
        n135 = call <vilib>:"compatOverwrite.vi"("overwrite (F)"=TRUE) -> ("overwrite?"=w478:T7)
        n136 = Bundle By Name(cluster=w501, "Drain Start"=w505, "Drain Stop"=w504, "Drain Step"=w503, "Drain Compliance"=w520, "Range mode"=w484, "Range"=w487) -> (w534:T5)
        n137 = call "4155C Output.vi"("VISA resource name in"=w490, "Gate"=w535, "Drain"=w534, "Timings"=w518, "error in (no error)"=w489, "SMU4"=w480, "sweep mode"=w511, "Panel controls"=w536) -> ("VD"=w471:dbl[], "Outparams"=w482:T8, "VISA Resource Name out"=w517:refnum<visa-resource-name>, "IS"=w470:dbl[], "ID"=w469:dbl[], "IG"=w468:dbl[], "error out"=w466:errorcluster, "SMU4"=w479:dbl[])  [unwired: 12 in]
        n138 = Unbundle By Name(w482) -> ("V2 Step"=w483:dbl, "V2 Start"=w481:dbl, "Number of points"=w463:i32)
        n139 = call "4155C Split array.vi"("Number of VAR2 steps"=w463, "Y2 data in"=w469, "X data in"=w471, "Y1 data in"=w470, "Y3 data in"=w468, "error in (no error)"=w466) -> ("Array of clusters"=w467:cluster{"Y data in":dbl[], "X data in":dbl[]}[], "error out"=w465:errorcluster)  [unwired: 1 in]
        n140 = local write "I vs Vd"(w467) -> ()
        n141 = call "4155C Config Chart Colours.vi"("Numeric"=w463, "XY Graph 2"=w464) -> ()  [unwired: 6 in]
        n142 = Open/Create/Replace File(file path (use dialog)=w521, error in=w465, operation (0:open)=w478) -> (refnum out=w531:refnum<file>, error out=w532:errorcluster)  [unwired: 3 in, 1 out]
        n143 = call "4155C Make Big 2d array.vi"("1D Var1"=w471, "1d IS"=w470, "1d ID"=w469, "1d IG"=w468, "1d SMU4"=w479, "SMU4"=w480, "VAR2 START"=w481, "Number of VAR2 steps"=w463, "VAR2 STEP"=w483, "VAR1 Name"="Vd", "Decimal places in header"=i8 1, "VAR2 Name"="Vg") -> ("Header array"=w527:string[], "Data array"=w528:dbl[][])  [unwired: 14 in]
        n144 = call "4155C Write array to file.vi"("Byte Stream File Refnum"=w531, "Header"=w527, "Data Array"=w528, "error in (no error)"=w532) -> ("dup refnum"=w529:refnum<file>, "error out"=w530:errorcluster)  [unwired: 1 in]
        n145 = Close File(refnum=w529, error in=w530) -> (error out=w516:errorcluster)  [unwired: 1 out]
      }
      frame "output-fpp" {
        n146 = Number To Decimal String(number=w544) -> (decimal integer string=w598:string)  [unwired: 1 in]
        n147 = Bundle By Name(cluster=w574, "Emergency Stop"=w601) -> (w611:T1)
        n148 = Delete From Array(array=w589, index=0 ("Index")) -> (deleted portion=w587:string, array with subset deleted=w586:string[])  [unwired: 1 in]
        n149 = VISA Write(VISA resource name=w565, write buffer=":PAGE:CHAN:MODE SWE;" ("write buffer (\"\")"), error in (no error)=w562) -> (VISA resource name out=w564:refnum<visa-resource-name>, error out=w563:errorcluster)  [unwired: 1 out]
        n150 = Concatenate Strings(w597, "-outputfpp-" ("Substring"), w598, w543, ".txt" ("Substring")) -> (w600:string)
        n151 = case shown="\"d\", Default" w587 {
          tunnel: [w612 w613] -> w585
          frame "s" {
            w612 = u16 0 items=["Single", "Double"] ("sweep mode")
          }
          frame "d", Default {
            w613 = u16 1 items=["Single", "Double"] ("sweep mode")
          }
        }
        n152 = Fract/Exp String To Number(string=w586) -> (number=w568:dbl[])  [unwired: 3 in, 1 out]
        n153 = String To Path(string=w600) -> (path=w596:path)
        n154 = Index Array(array=w568, index #1=0 ("Index")) -> (element #1=w584:dbl, element #2=w583:dbl, element #3=w582:dbl)  [unwired: 2 in]
        n155 = Delete From Array(array=w568, length=3 ("Length"), index=0 ("Index")) -> (array with subset deleted=w567:dbl[])  [unwired: 1 out]
        n156 = Bundle By Name(cluster=w576, "Gate Start"=w584, "Gate Stop"=w583, "Gate Step (linear only)"=w582, "Gate Compliance"=w594, "Range mode"=w560, "Range"=w559) -> (w610:T4)
        n157 = Index Array(array=w567, index #1=0 ("Index")) -> (element #1=w579:dbl, element #2=w578:dbl, element #3=w577:dbl)  [unwired: 2 in]
        n158 = call <vilib>:"compatOverwrite.vi"("overwrite (F)"=TRUE) -> ("overwrite?"=w548:T7)
        n159 = Bundle By Name(cluster=w575, "Drain Start"=w579, "Drain Stop"=w578, "Drain Step"=w577, "Drain Compliance"=w595, "Range mode"=w558, "Range"=w561) -> (w609:T5)
        n160 = call "4155C Output-FPP.vi"("VISA resource name in"=w564, "Gate"=w610, "Drain"=w609, "Timings"=w593, "error in (no error)"=w563, "sweep mode"=w585, "Panel controls"=w611) -> ("VD"=w553:dbl[], "Outparams"=w556:T8, "VISA Resource Name out"=w591:refnum<visa-resource-name>, "Vprobe2"=w552:dbl[], "ID"=w551:dbl[], "IG"=w550:dbl[], "Vprobe1"=w549:dbl[], "error out"=w592:errorcluster)  [unwired: 13 in]
        n161 = Unbundle By Name(w556) -> ("V2 Step"=w557:dbl, "V2 Start"=w555:dbl, "Number of points"=w554:i32)
        n162 = Open/Create/Replace File(file path (use dialog)=w596, error in=w592, operation (0:open)=w548) -> (refnum out=w606:refnum<file>, error out=w607:errorcluster)  [unwired: 3 in, 1 out]
        n163 = call "4155C Make Big 2d array FPP.vi"("1D Var1"=w553, "1d ID"=w551, "1d Vp2"=w552, "1d IG"=w550, "1d Vp1"=w549, "VAR2 START"=w555, "Number of VAR2 steps"=w554, "VAR2 STEP"=w557, "VAR1 Name"="Vd", "Decimal places in header"=i8 1, "VAR2 Name"="Vg") -> ("Header array"=w602:string[], "Data array"=w603:dbl[][])  [unwired: 15 in]
        n164 = call "4155C Write array to file.vi"("Byte Stream File Refnum"=w606, "Header"=w602, "Data Array"=w603, "error in (no error)"=w607) -> ("dup refnum"=w604:refnum<file>, "error out"=w605:errorcluster)  [unwired: 1 in]
        n165 = Close File(refnum=w604, error in=w605) -> (error out=w590:errorcluster)  [unwired: 1 out]
      }
      frame "itime" {
        n166 = Delete From Array(array=w631, index=0 ("Index")) -> (deleted portion=w632:string)  [unwired: 1 in, 1 out]
        n167 = case shown="\"l\"" w632 {
          tunnel: w630 -> [w636 w638 w641]
          tunnel: [w635 w637 w640] -> w623
          frame "s" {
            w634 = u32 0 items=["short  ", "medium  ", "long  "] ("integration time 2")
            n168 = Bundle By Name(cluster=w636, "integration time"=w634) -> (w635:T6)
          }
          frame "m", Default {
            w639 = u32 1 items=["short  ", "medium  ", "long  "] ("integration time 2")
            n169 = Bundle By Name(cluster=w638, "integration time"=w639) -> (w637:T6)
          }
          frame "l" {
            w642 = u32 2 items=["short  ", "medium  ", "long  "] ("integration time 2")
            n170 = Bundle By Name(cluster=w641, "integration time"=w642) -> (w640:T6)
          }
        }
      }
      frame "pulsed" {
        n171 = Delete From Array(array=w661, index=0 ("Index")) -> (deleted portion=w662:string, array with subset deleted=w649:string[])  [unwired: 1 in]
        n172 = case shown="\"on\", Default" w662 {
          tunnel: w660 -> [w672 w675]
          tunnel: [w671 w674] -> w653
          tunnel: w649 -> [w669 _]
          frame "on", Default {
            w670 = u16 1 items=["Continuous", "Pulsed"] ("sweep method")
            n173 = Fract/Exp String To Number(string=w669) -> (number=w667:dbl[])  [unwired: 3 in, 1 out]
            n174 = Index Array(array=w667, index #1=0 ("Index")) -> (element #1=w666:dbl, element #2=w665:dbl, element #3=w664:dbl)  [unwired: 2 in]
            n175 = Bundle By Name(cluster=w672, "sweep method"=w670, "Pulse period"=w666, "Base voltage"=w665, "Pulse width"=w664) -> (w671:T6)
          }
          frame "off" {
            w673 = u16 0 items=["Continuous", "Pulsed"] ("sweep method")
            n176 = Bundle By Name(cluster=w675, "sweep method"=w673) -> (w674:T6)
          }
        }
      }
      frame "gaterangemode" {
        n177 = Delete From Array(array=w692, index=0 ("Index")) -> (deleted portion=w693:string)  [unwired: 1 in, 1 out]
        n178 = case shown="\"f\"" w693 {
          tunnel: [w695 w696 w697] -> w682
          frame "a", Default {
            w695 = u16 0 items=["Auto", "Limited", "Fixed"] ("Gate Range\nmode 2")
          }
          frame "f" {
            w696 = u16 2 items=["Auto", "Limited", "Fixed"] ("Gate Range\nmode 2")
          }
          frame "l" {
            w697 = u16 1 items=["Auto", "Limited", "Fixed"] ("Gate Range\nmode 2")
          }
        }
      }
      frame "gaterange" {
        (unwired) u8 11 items=["10fA  ", "100fA  ", "1nA  ", "10nA", "100nA", "1uA", "10uA", "100uA", "1mA", "10mA", "100mA", "1A"] ("Gate Range 2")
        n179 = Delete From Array(array=w721, index=0 ("Index")) -> (deleted portion=w711:string)  [unwired: 1 in, 1 out]
        n180 = Scan Value(string=w711, format string="") -> (value=w709:dbl)  [unwired: 1 in, 1 out]
        n181 = Logarithm Base 10(1:w709) -> (0:w708:dbl)
        n182 = Round To Nearest(number=w708) -> (nearest integer value=w707:dbl)
        n183 = Add(x=w707, y=11.0) -> (x+y=w705:dbl)
        n184 = To Unsigned Byte Integer(number=w705) -> (unsigned 8bit integer=w704:u8)
      }
      frame "drainrange" {
        (unwired) u8 11 items=["10fA  ", "100fA  ", "1nA  ", "10nA", "100nA", "1uA", "10uA", "100uA", "1mA", "10mA", "100mA", "1A"] ("Gate Range 2")
        n185 = Delete From Array(array=w746, index=0 ("Index")) -> (deleted portion=w737:string)  [unwired: 1 in, 1 out]
        n186 = Scan Value(string=w737, format string="") -> (value=w735:dbl)  [unwired: 1 in, 1 out]
        n187 = Logarithm Base 10(1:w735) -> (0:w734:dbl)
        n188 = Round To Nearest(number=w734) -> (nearest integer value=w733:dbl)
        n189 = Add(x=w733, y=11.0) -> (x+y=w731:dbl)
        n190 = To Unsigned Byte Integer(number=w731) -> (unsigned 8bit integer=w730:u8)
      }
      frame "drainrangemode" {
        n191 = Delete From Array(array=w764, index=0 ("Index")) -> (deleted portion=w765:string)  [unwired: 1 in, 1 out]
        n192 = case shown="\"f\"" w765 {
          tunnel: [w767 w768 w769] -> w754
          frame "a", Default {
            w767 = u16 0 items=["Auto", "Limited", "Fixed"] ("Gate Range\nmode 2")
          }
          frame "f" {
            w768 = u16 2 items=["Auto", "Limited", "Fixed"] ("Gate Range\nmode 2")
          }
          frame "l" {
            w769 = u16 1 items=["Auto", "Limited", "Fixed"] ("Gate Range\nmode 2")
          }
        }
      }
      frame "Error", Default {
      }
      frame "logfile" {
        n193 = Number To Decimal String(number=w792) -> (decimal integer string=w827:string)  [unwired: 1 in]
        n194 = Concatenate Strings(w826, "logfile" ("Substring"), w827, w790, ".txt" ("Substring")) -> (w824:string)
        n195 = String To Path(string=w824) -> (path=w797:path)
        n196 = Unbundle(w823) -> ("integration time"=w822:u32, "Short/Long integration time"=w821:dbl, "hold time (sec)"=w820:dbl, "delay time (sec)"=w819:dbl, "Step Time (0 disables)"=w818:dbl, "sweep method"=w817:u16, "Pulse period"=w816:dbl, "Base voltage"=w815:dbl, "Pulse width"=w814:dbl)
        n197 = Build Array(w822, w821, w820, w819, w818, w817, w816, w815, w814, w808, w809, w810, w811, w812, w813) -> (w801:dbl[])
        n198 = Insert Into Array(array=dbl[][] [] ("Input Array"), new element=w801) -> (w800:dbl[][])  [unwired: 2 in]
        n199 = call <vilib>:"compatOverwrite.vi"("overwrite (F)"=TRUE) -> ("overwrite?"=w795:T7)
        n200 = Open/Create/Replace File(file path (use dialog)=w797, error in=w799, operation (0:open)=w795) -> (refnum out=w805:refnum<file>, error out=w804:errorcluster)  [unwired: 3 in, 1 out]
        n201 = call "4155C Write array to file.vi"("Byte Stream File Refnum"=w805, "Header"=string[] ["Int Time", "Short/Long Itime", "Hold time", "Delay time", "Step time", "Sweep method", "Pulse period", "Base Voltage", "Pulse width", "Drain compliance", "Gate compliance", "Gate range mode", "Gate range", "S/D range mode", "S/D range"], "Data Array"=w800, "error in (no error)"=w804) -> ("dup refnum"=w807:refnum<file>, "error out"=w806:errorcluster)  [unwired: 1 in]
        n202 = Close File(refnum=w807, error in=w806) -> (error out=w798:errorcluster)  [unwired: 1 out]
      }
      frame "sample" {
        n203 = Number To Decimal String(number=w835) -> (decimal integer string=w883:string)  [unwired: 1 in]
        n204 = Fract/Exp String To Number(string=w880) -> (number=w841:dbl[])  [unwired: 3 in, 1 out]
        n205 = Concatenate Strings(w858, "-sample-" ("Substring"), w883, w833, ".txt" ("Substring")) -> (w881:string)
        n206 = String To Path(string=w881) -> (path=w862:path)
        n207 = Index Array(array=w841, index=0 ("Index")) -> (element=w878:dbl)
        n208 = Index Array(array=w841, index=2 ("Index")) -> (element=w874:dbl)
        n209 = Index Array(array=w841, index=3 ("Index")) -> (element=w843:dbl)
        n210 = Index Array(array=w841, index=4 ("Index")) -> (element=w840:dbl)
        n211 = call "4155C Config Sampling Measurements.vi"("Sampling interval"=w840, "Sample time"=w843, "Display on/off"=TRUE, "Timings"=w849, "Num Points"=w874, "error in (no error)"=w885, "Drain Compliance"=w884, "Gate Compliance"=w859, "VISA session"=w886) -> ("error out"=w887:errorcluster, "dup VISA resource name"=w888:refnum<visa-resource-name>)  [unwired: 1 in]
        n212 = Index Array(array=w841, index=1 ("Index")) -> (element=w875:dbl)
        n213 = call "4155C Take Sample.vi"("Emergency Stop"=w855, "error in (no error)"=w887, "Vd"=w875, "Vg"=w878, "VISA resource name in"=w888) -> ("error out"=w853:errorcluster, "Id"=w890:dbl[], "Ig"=w864:dbl[], "VISA Resource Name out"=w851:refnum<visa-resource-name>, "Is"=w889:dbl[], "Time"=w868:dbl[])  [unwired: 1 in]
        n214 = Insert Into Array(array=dbl[][] [] ("Input Array"), new element=w868) -> (w867:dbl[][])  [unwired: 2 in]
        n215 = Insert Into Array(array=w867, new element=w864) -> (w866:dbl[][])  [unwired: 2 in]
        n216 = Insert Into Array(array=w866, new element=w890) -> (w865:dbl[][])  [unwired: 2 in]
        n217 = VISA Write(VISA resource name=w851, write buffer=":DISP ON" ("write buffer (\"\")"), error in (no error)=w853) -> (VISA resource name out=w850:refnum<visa-resource-name>, error out=w852:errorcluster)  [unwired: 1 out]
        n218 = Insert Into Array(array=w865, new element=w889) -> (w857:dbl[][])  [unwired: 2 in]
        n219 = Transpose 2D Array(2D array=w857) -> (transposed array=w856:dbl[][])
        n220 = call <vilib>:"compatOverwrite.vi"("overwrite (F)"=TRUE) -> ("overwrite?"=w838:T7)
        n221 = Open/Create/Replace File(file path (use dialog)=w862, error in=w852, operation (0:open)=w838) -> (refnum out=w871:refnum<file>, error out=w870:errorcluster)  [unwired: 3 in, 1 out]
        n222 = call "4155C Write array to file.vi"("Byte Stream File Refnum"=w871, "Header"=string[] ["Time /s", "Ig /A", "Id /A", "Is /A"], "Data Array"=w856, "error in (no error)"=w870) -> ("dup refnum"=w873:refnum<file>, "error out"=w872:errorcluster)  [unwired: 1 in]
        n223 = Close File(refnum=w873, error in=w872) -> (error out=w860:errorcluster)  [unwired: 1 out]
      }
      frame "samplei" {
        n224 = Number To Decimal String(number=w896) -> (decimal integer string=w948:string)  [unwired: 1 in]
        n225 = Fract/Exp String To Number(string=w945) -> (number=w912:dbl[])  [unwired: 3 in, 1 out]
        n226 = Concatenate Strings(w927, "-samplei-" ("Substring"), w948, w895, ".txt" ("Substring")) -> (w946:string)
        n227 = String To Path(string=w946) -> (path=w930:path)
        n228 = Index Array(array=w912, index=4 ("Index")) -> (element=w906:dbl)
        n229 = Index Array(array=w912, index=3 ("Index")) -> (element=w907:dbl)
        n230 = Index Array(array=w912, index=1 ("Index")) -> (element=w909:dbl)
        n231 = Index Array(array=w912, index=0 ("Index")) -> (element=w910:dbl)
        n232 = Index Array(array=w912, index=2 ("Index")) -> (element=w908:dbl)
        n233 = call "4155C Config SamplingI Measurements.vi"("Sample time"=w908, "Display on/off"=TRUE, "Timings"=w919, "Num Points"=w909, "error in (no error)"=w950, "Sampling interval"=w907, "VISA session"=w951) -> ("error out"=w952:errorcluster, "dup VISA resource name"=w953:refnum<visa-resource-name>)  [unwired: 3 in]
        n234 = call "4155C Take SampleI.vi"("Emergency Stop"=w924, "error in (no error)"=w952, "Idg 2"=w910, "Vdg compliance 2"=w906, "VISA resource name in"=w953) -> ("error out"=w922:errorcluster, "Idg"=w955:dbl[], "Vdg"=w932:dbl[], "VISA Resource Name out"=w920:refnum<visa-resource-name>, "Is"=w954:dbl[], "Time"=w936:dbl[])  [unwired: 1 in]
        n235 = Insert Into Array(array=dbl[][] [] ("Input Array"), new element=w936) -> (w935:dbl[][])  [unwired: 2 in]
        n236 = Insert Into Array(array=w935, new element=w932) -> (w934:dbl[][])  [unwired: 2 in]
        n237 = Insert Into Array(array=w934, new element=w955) -> (w933:dbl[][])  [unwired: 2 in]
        n238 = VISA Write(VISA resource name=w920, write buffer=":DISP ON" ("write buffer (\"\")"), error in (no error)=w922) -> (VISA resource name out=w905:refnum<visa-resource-name>, error out=w921:errorcluster)  [unwired: 1 out]
        n239 = Insert Into Array(array=w933, new element=w954) -> (w926:dbl[][])  [unwired: 2 in]
        n240 = Transpose 2D Array(2D array=w926) -> (transposed array=w925:dbl[][])
        n241 = call <vilib>:"compatOverwrite.vi"("overwrite (F)"=TRUE) -> ("overwrite?"=w900:T7)
        n242 = Open/Create/Replace File(file path (use dialog)=w930, error in=w921, operation (0:open)=w900) -> (refnum out=w939:refnum<file>, error out=w938:errorcluster)  [unwired: 3 in, 1 out]
        n243 = call "4155C Write array to file.vi"("Byte Stream File Refnum"=w939, "Header"=string[] ["Time /s", "Vdg /V", "Idg /A", "Is /A"], "Data Array"=w925, "error in (no error)"=w938) -> ("dup refnum"=w941:refnum<file>, "error out"=w940:errorcluster)  [unwired: 1 in]
        n244 = Close File(refnum=w941, error in=w940) -> (error out=w903:errorcluster)  [unwired: 1 out]
        n245 = VISA Write(VISA resource name=w905, write buffer=";:PAGE:SCON:STAN OFF;:PAGE:CHAN:VSU2:DIS;" ("write buffer (\"\")"), error in (no error)=w903) -> (VISA resource name out=w901:refnum<visa-resource-name>, error out=w902:errorcluster)  [unwired: 1 out]
      }
      frame "#" {
        n246 = VISA Write(VISA resource name=w966, write buffer=":DISP ON" ("write buffer (\"\")"), error in (no error)=w965) -> (VISA resource name out=w964:refnum<visa-resource-name>, error out=w963:errorcluster)  [unwired: 1 out]
      }
      frame "stressV" {
        n247 = Number To Decimal String(number=w980) -> (decimal integer string=w1021:string)  [unwired: 1 in]
        n248 = Fract/Exp String To Number(string=w1018) -> (number=w991:dbl[])  [unwired: 3 in, 1 out]
        n249 = Concatenate Strings(w1005, "-stressV-" ("Substring"), w1021, w979, ".txt" ("Substring")) -> (w1019:string)
        n250 = String To Path(string=w1019) -> (path=w1009:path)
        n251 = Index Array(array=w991, index=3 ("Index")) -> (element=w988:dbl)
        n252 = Index Array(array=w991, index=1 ("Index")) -> (element=w986:dbl)
        n253 = Index Array(array=w991, index=0 ("Index")) -> (element=w985:dbl)
        n254 = Index Array(array=w991, index=4 ("Index")) -> (element=w990:dbl)
        n255 = Index Array(array=w991, index=2 ("Index")) -> (element=w987:dbl)
        n256 = call "4155C Config V Stress.vi"("VISA session"=w1024, "ID compliance"=w988, "VD"=w986, "VG"=w985, "IG compliance"=w987, "error in (no error)"=w1023, "Display on/off"=TRUE) -> ("dup VISA resource name"=w1026:refnum<visa-resource-name>, "error out"=w1025:errorcluster)
        n257 = call "4155C Apply Stress.vi"("error in (no error)"=w1025, "Duration"=w990, "Emergency Stop"=w1004, "VISA resource name in"=w1026) -> ("error out"=w1002:errorcluster, "VISA Resource Name out"=w1000:refnum<visa-resource-name>)
        n258 = VISA Write(VISA resource name=w1000, write buffer=":DISP ON" ("write buffer (\"\")"), error in (no error)=w1002) -> (VISA resource name out=w999:refnum<visa-resource-name>, error out=w1001:errorcluster)  [unwired: 1 out]
        n259 = call <vilib>:"compatOverwrite.vi"("overwrite (F)"=TRUE) -> ("overwrite?"=w984:T7)
        n260 = Open/Create/Replace File(file path (use dialog)=w1009, error in=w1001, operation (0:open)=w984) -> (refnum out=w1012:refnum<file>, error out=w1011:errorcluster)  [unwired: 3 in, 1 out]
        n261 = call "4155C Write array to file.vi"("Byte Stream File Refnum"=w1012, "Header"=string[] ["V stress completed successfully", ""], "error in (no error)"=w1011) -> ("dup refnum"=w1014:refnum<file>, "error out"=w1013:errorcluster)  [unwired: 2 in]
        n262 = Close File(refnum=w1014, error in=w1013) -> (error out=w1007:errorcluster)  [unwired: 1 out]
      }
      frame "stressI" {
        n263 = Number To Decimal String(number=w1032) -> (decimal integer string=w1069:string)  [unwired: 1 in]
        n264 = Fract/Exp String To Number(string=w1066) -> (number=w1041:dbl[])  [unwired: 3 in, 1 out]
        n265 = Concatenate Strings(w1053, "-stressI-" ("Substring"), w1069, w1031, ".txt" ("Substring")) -> (w1067:string)
        n266 = String To Path(string=w1067) -> (path=w1057:path)
        n267 = Index Array(array=w1041, index=1 ("Index")) -> (element=w1037:dbl)
        n268 = Index Array(array=w1041, index=0 ("Index")) -> (element=w1038:dbl)
        n269 = call "4155C Config I Stress.vi"("VISA session"=w1072, "IDG"=w1038, "VDG compliance"=w1037, "error in (no error)"=w1071, "Display on/off"=TRUE) -> ("dup VISA resource name"=w1074:refnum<visa-resource-name>, "error out"=w1073:errorcluster)
        n270 = Index Array(array=w1041, index=2 ("Index")) -> (element=w1039:dbl)
        n271 = call "4155C Apply Stress.vi"("error in (no error)"=w1073, "Duration"=w1039, "Emergency Stop"=w1052, "VISA resource name in"=w1074) -> ("error out"=w1050:errorcluster, "VISA Resource Name out"=w1048:refnum<visa-resource-name>)
        n272 = VISA Write(VISA resource name=w1048, write buffer=":DISP ON" ("write buffer (\"\")"), error in (no error)=w1050) -> (VISA resource name out=w1047:refnum<visa-resource-name>, error out=w1049:errorcluster)  [unwired: 1 out]
        n273 = call <vilib>:"compatOverwrite.vi"("overwrite (F)"=TRUE) -> ("overwrite?"=w1036:T7)
        n274 = Open/Create/Replace File(file path (use dialog)=w1057, error in=w1049, operation (0:open)=w1036) -> (refnum out=w1060:refnum<file>, error out=w1059:errorcluster)  [unwired: 3 in, 1 out]
        n275 = call "4155C Write array to file.vi"("Byte Stream File Refnum"=w1060, "Header"=string[] ["I stress completed successfully", ""], "error in (no error)"=w1059) -> ("dup refnum"=w1062:refnum<file>, "error out"=w1061:errorcluster)  [unwired: 2 in]
        n276 = Close File(refnum=w1062, error in=w1061) -> (error out=w1055:errorcluster)  [unwired: 1 out]
      }
      frame "vsu2pulse" {
        n277 = Number To Decimal String(number=w1080) -> (decimal integer string=w1115:string)  [unwired: 1 in]
        n278 = Fract/Exp String To Number(string=w1112) -> (number=w1088:dbl[])  [unwired: 3 in, 1 out]
        n279 = Concatenate Strings(w1100, "-vsu2-" ("Substring"), w1115, w1079, ".txt" ("Substring")) -> (w1113:string)
        n280 = String To Path(string=w1113) -> (path=w1104:path)
        n281 = Index Array(array=w1088, index=1 ("Index")) -> (element=w1087:dbl)
        n282 = Index Array(array=w1088, index=0 ("Index")) -> (element=w1085:dbl)
        n283 = call "4155C Config VSU2 Stress.vi"("error in (no error)"=w1117, "VSU2"=w1085, "Display on/off"=TRUE, "VISA session"=w1118) -> ("error out"=w1119:errorcluster, "dup VISA resource name"=w1120:refnum<visa-resource-name>)
        n284 = call "4155C Apply Stress.vi"("error in (no error)"=w1119, "Duration"=w1087, "Emergency Stop"=w1099, "VISA resource name in"=w1120) -> ("error out"=w1097:errorcluster, "VISA Resource Name out"=w1095:refnum<visa-resource-name>)
        n285 = VISA Write(VISA resource name=w1095, write buffer=":DISP ON" ("write buffer (\"\")"), error in (no error)=w1097) -> (VISA resource name out=w1094:refnum<visa-resource-name>, error out=w1096:errorcluster)  [unwired: 1 out]
        n286 = call <vilib>:"compatOverwrite.vi"("overwrite (F)"=TRUE) -> ("overwrite?"=w1084:T7)
        n287 = Open/Create/Replace File(file path (use dialog)=w1104, error in=w1096, operation (0:open)=w1084) -> (refnum out=w1107:refnum<file>, error out=w1106:errorcluster)  [unwired: 3 in, 1 out]
        n288 = call "4155C Write array to file.vi"("Byte Stream File Refnum"=w1107, "Header"=string[] ["VSU2 pulse completed successfully", ""], "error in (no error)"=w1106) -> ("dup refnum"=w1109:refnum<file>, "error out"=w1108:errorcluster)  [unwired: 2 in]
        n289 = Close File(refnum=w1109, error in=w1108) -> (error out=w1102:errorcluster)  [unwired: 1 out]
      }
      frame "sample-fpp" {
        w1137 = string[] ["Time /s", "Id VgVd /A", "Ig VgVd /A", "Vp1 VgVd /V", "Vp2 VgVd /V"] ("Header")
        w1141 = "%d" ("format string")
        n290 = Number To Decimal String(number=w1126) -> (decimal integer string=w1189:string)  [unwired: 1 in]
        n291 = Fract/Exp String To Number(string=w1186) -> (number=w1174:dbl[])  [unwired: 3 in, 1 out]
        n292 = Concatenate Strings(w1180, "-samplefpp-" ("Substring"), w1189, w1125, ".txt" ("Substring")) -> (w1187:string)
        n293 = String To Path(string=w1187) -> (path=w1149:path)
        n294 = Index Array(array=w1174, index=0 ("Index")) -> (element=w1135:dbl)
        n295 = Index Array(array=w1174, index=1 ("Index")) -> (element=w1134:dbl)
        n296 = Index Array(array=w1174, index=2 ("Index")) -> (element=w1182:dbl)
        n297 = Index Array(array=w1174, index=3 ("Index")) -> (element=w1172:dbl)
        n298 = call "4155C Config Sampling Measurements FPP.vi"("VISA session"=w1192, "Num Points"=w1182, "Vg"=w1135, "Display on/off"=TRUE, "Gate Compliance"=w1181, "Drain Compliance"=w1190, "Standby"="Standby", "error in (no error)"=w1191, "Timings"=w1179, "Vd"=w1134, "Sample time"=w1172) -> ("dup VISA resource name"=w1151:refnum<visa-resource-name>, "error out"=w1150:errorcluster)  [unwired: 3 in]
        n299 = Number To Decimal String(number=w1135) -> (decimal integer string=w1161:string)  [unwired: 1 in]
        n300 = call "4155C Take Sample FPP.vi"("VISA resource name in"=w1151, "error in (no error)"=w1150, "Emergency Stop"=w1152) -> ("Time"=w1156:dbl[], "Vp1"=w1166:dbl[], "VISA Resource Name out"=w1132:refnum<visa-resource-name>, "Ig"=w1154:dbl[], "Id"=w1155:dbl[], "Vp2"=w1164:dbl[], "error out"=w1153:errorcluster)  [unwired: 10 in]
        n301 = Insert Into Array(array=dbl[][] [] ("Input Array"), new element=w1156) -> (w1170:dbl[][])  [unwired: 2 in]
        n302 = Number To Decimal String(number=w1134) -> (decimal integer string=w1159:string)  [unwired: 1 in]
        n303 = Insert Into Array(array=w1170, new element=w1155) -> (w1169:dbl[][])  [unwired: 2 in]
        n304 = Concatenate Strings("(Vg = " ("Substring"), w1161, "V, Vd = " ("Substring"), w1159, "V)" ("Substring")) -> (w1157:string)
        n305 = Insert Into Array(array=w1169, new element=w1154) -> (w1168:dbl[][])  [unwired: 2 in]
        n306 = Insert Into Array(array=w1168, new element=w1166) -> (w1165:dbl[][])  [unwired: 2 in]
        n307 = Insert Into Array(array=w1165, new element=w1164) -> (w1133:dbl[][])  [unwired: 2 in]
        n308 = call <vilib>:"compatOverwrite.vi"("overwrite (F)"=TRUE) -> ("overwrite?"=w1130:T7)
        n309 = Open/Create/Replace File(file path (use dialog)=w1149, error in=w1153, operation (0:open)=w1130) -> (refnum out=w1146:refnum<file>, error out=w1147:errorcluster)  [unwired: 3 in, 1 out]
        n310 = Array To Spreadsheet String(array=w1137, 3:w1141) -> (spreadsheet string=w1143:string)  [unwired: 1 in]
        n311 = Transpose 2D Array(2D array=w1133) -> (transposed array=w1163:dbl[][])
        n312 = Search and Replace String(replace all?=TRUE ("replace all? (F)"), input string=w1143, search string="VgVd", replace string=w1157) -> (result string=w1139:string)  [unwired: 4 in, 3 out]
        n313 = Spreadsheet String To Array(format string=w1141, spreadsheet string=w1139, array type (2D Dbl)=w1137) -> (array=w1138:string[])  [unwired: 1 in]
        n314 = call "4155C Write array to file.vi"("Byte Stream File Refnum"=w1146, "Header"=w1138, "Data Array"=w1163, "error in (no error)"=w1147) -> ("dup refnum"=w1144:refnum<file>, "error out"=w1145:errorcluster)  [unwired: 1 in]
        n315 = Close File(refnum=w1144, error in=w1145) -> (error out=w1131:errorcluster)  [unwired: 1 out]
      }
      frame "resample-fpp" {
        w1211 = string[] ["Time /s", "Id VgVd /A", "Ig VgVd /A", "Vp1 VgVd /V", "Vp2 VgVd /V"] ("Header")
        w1215 = "%d" ("format string")
        n316 = Number To Decimal String(number=w1197) -> (decimal integer string=w1255:string)  [unwired: 1 in]
        n317 = Fract/Exp String To Number(string=w1252) -> (number=w1204:dbl[])  [unwired: 3 in, 1 out]
        n318 = Concatenate Strings(w1248, "-resamplefpp-" ("Substring"), w1255, w1198, ".txt" ("Substring")) -> (w1253:string)
        n319 = String To Path(string=w1253) -> (path=w1223:path)
        n320 = Index Array(array=w1204, index=0 ("Index")) -> (element=w1210:dbl)
        n321 = Index Array(array=w1204, index=1 ("Index")) -> (element=w1209:dbl)
        n322 = Number To Decimal String(number=w1210) -> (decimal integer string=w1233:string)  [unwired: 1 in]
        n323 = call "4155C Take Sample FPP.vi"("VISA resource name in"=w1206, "error in (no error)"=w1205, "Emergency Stop"=w1224) -> ("Time"=w1228:dbl[], "Vp1"=w1238:dbl[], "VISA Resource Name out"=w1208:refnum<visa-resource-name>, "Ig"=w1226:dbl[], "Id"=w1227:dbl[], "Vp2"=w1236:dbl[], "error out"=w1225:errorcluster)  [unwired: 10 in]
        n324 = Insert Into Array(array=dbl[][] [] ("Input Array"), new element=w1228) -> (w1242:dbl[][])  [unwired: 2 in]
        n325 = Number To Decimal String(number=w1209) -> (decimal integer string=w1231:string)  [unwired: 1 in]
        n326 = Insert Into Array(array=w1242, new element=w1227) -> (w1241:dbl[][])  [unwired: 2 in]
        n327 = Concatenate Strings("(Vg = " ("Substring"), w1233, "V, Vd = " ("Substring"), w1231, "V)" ("Substring")) -> (w1229:string)
        n328 = Insert Into Array(array=w1241, new element=w1226) -> (w1240:dbl[][])  [unwired: 2 in]
        n329 = Insert Into Array(array=w1240, new element=w1238) -> (w1237:dbl[][])  [unwired: 2 in]
        n330 = Insert Into Array(array=w1237, new element=w1236) -> (w1203:dbl[][])  [unwired: 2 in]
        n331 = call <vilib>:"compatOverwrite.vi"("overwrite (F)"=TRUE) -> ("overwrite?"=w1202:T7)
        n332 = Open/Create/Replace File(file path (use dialog)=w1223, error in=w1225, operation (0:open)=w1202) -> (refnum out=w1220:refnum<file>, error out=w1221:errorcluster)  [unwired: 3 in, 1 out]
        n333 = Array To Spreadsheet String(array=w1211, 3:w1215) -> (spreadsheet string=w1217:string)  [unwired: 1 in]
        n334 = Transpose 2D Array(2D array=w1203) -> (transposed array=w1235:dbl[][])
        n335 = Search and Replace String(replace all?=TRUE ("replace all? (F)"), input string=w1217, search string="VgVd", replace string=w1229) -> (result string=w1213:string)  [unwired: 4 in, 3 out]
        n336 = Spreadsheet String To Array(format string=w1215, spreadsheet string=w1213, array type (2D Dbl)=w1211) -> (array=w1212:string[])  [unwired: 1 in]
        n337 = call "4155C Write array to file.vi"("Byte Stream File Refnum"=w1220, "Header"=w1212, "Data Array"=w1235, "error in (no error)"=w1221) -> ("dup refnum"=w1218:refnum<file>, "error out"=w1219:errorcluster)  [unwired: 1 in]
        n338 = Close File(refnum=w1218, error in=w1219) -> (error out=w1207:errorcluster)  [unwired: 1 out]
      }
      frame "serial" {
        n339 = local read "Enable Termination\nChar (T)"() -> (w1269:bool)
        n340 = local read "Termination char\n(0xA = '\\n' = LF)\n(0xD = '\\r' = CR)"() -> (w1268:u8)
        n341 = Index Array(array=w1276, index=0 ("Index")) -> (element=w1275:string)
        n342 = local read "parity"() -> (w1259:u16)
        n343 = local read "Delay before read (ms)"() -> (w1270:u32)
        n344 = local read "byte count"() -> (w1267:u32)
        n345 = local read "Timeout (ms)"() -> (w1266:u32)
        n346 = local read "VISA resource name"() -> (w1263:refnum<visa-resource-name>)
        n347 = local read "baud rate"() -> (w1262:u32)
        n348 = local read "Serial End Mode for Reads"() -> (w1261:u16)
        n349 = local read "data bits"() -> (w1260:u16)
        n350 = local read "stop bits"() -> (w1265:u16)
        n351 = local read "flow control"() -> (w1264:u16)
        n352 = call "Serial write and read v0.5.vi"("Delay before read (ms)"=w1270, "Termination char\n(0xA = '\\n' = LF)\n(0xD = '\\r' = CR)"=w1268, "Enable Termination\nChar (T)"=w1269, "parity"=w1259, "stop bits"=w1265, "string to write"=w1275, "flow control"=w1264, "byte count"=w1267, "Serial Settings:Serial End Mode for Reads"=w1261, "Timeout (ms)"=w1266, "error in (no error)"=w1281, "VISA resource name"=w1263, "baud rate"=w1262, "data bits"=w1260) -> ("Serial port output"=w1271:string, "error out"=w1280:errorcluster)
        n353 = Build Array (concatenate)(w1271, w1272) -> (w1273:string[])
      }
      frame "pump" {
        n354 = local read "Enable Termination\nChar (T)"() -> (w1312:bool)
        n355 = local read "Termination char\n(0xA = '\\n' = LF)\n(0xD = '\\r' = CR)"() -> (w1311:u8)
        n356 = Index Array(array=w1321, index=0 ("Index")) -> (element=w1320:string)
        n357 = local read "flow control"() -> (w1307:u16)
        n358 = local read "stop bits"() -> (w1308:u16)
        n359 = local read "parity"() -> (w1302:u16)
        n360 = local read "Delay before read (ms)"() -> (w1313:u32)
        n361 = local read "byte count"() -> (w1310:u32)
        n362 = local read "Timeout (ms)"() -> (w1309:u32)
        n363 = local read "VISA resource name"() -> (w1306:refnum<visa-resource-name>)
        n364 = local read "baud rate"() -> (w1305:u32)
        n365 = local read "Serial End Mode for Reads"() -> (w1304:u16)
        n366 = Number To Decimal String(number=w1316) -> (decimal integer string=w1315:string)  [unwired: 1 in]
        n367 = local read "data bits"() -> (w1303:u16)
        n368 = call "SPM Pump v0.3.vi"("Termination char\n(0xA = '\\n' = LF)\n(0xD = '\\r' = CR)"=w1311, "Enable Termination\nChar (T)"=w1312, "Timeout (ms)"=w1309, "Serial Settings:Serial End Mode for Reads"=w1304, "byte count"=w1310, "Delay before read (ms)"=w1313, "Time <input>"=w1315, "error in (no error)"=w1326, "Serial port input"=w1320, "VISA resource name"=w1306, "parity"=w1302, "baud rate"=w1305, "stop bits"=w1308, "data bits"=w1303, "flow control"=w1307) -> ("Valve position"=w1295:string, "Absolute plunger position"=w1300:string, "Serial port output"=w1314:string, "error out"=w1325:errorcluster)  [unwired: 5 in, 4 out]
        n369 = Decimal String To Number(string=w1300) -> (number=w1299:i32)  [unwired: 2 in, 1 out]
        n370 = Decimal String To Number(string=w1295) -> (number=w1293:i32)  [unwired: 2 in, 1 out]
        n371 = Build Array (concatenate)(w1291, w1293) -> (w1292:i32[])
        n372 = Build Array (concatenate)(w1297, w1299) -> (w1298:i32[])
        n373 = call "4155C Split array.vi"("X data in"=w1296, "Y1 data in"=w1292) -> ("Array of clusters"=w1294:cluster{"Y data in":dbl[], "X data in":dbl[]}[])  [unwired: 5 in, 1 out]
        n374 = local write "Valve position vs time"(w1294) -> ()
        n375 = call "4155C Split array.vi"("X data in"=w1296, "Y1 data in"=w1298) -> ("Array of clusters"=w1301:cluster{"Y data in":dbl[], "X data in":dbl[]}[])  [unwired: 5 in, 1 out]
        n376 = local write "Absolute plunger position vs time"(w1301) -> ()
        n377 = Build Array (concatenate)(w1314, w1317) -> (w1318:string[])
      }
    }
    n378 = Build Array(w86, w85, w79, w53) -> (w84:dbl[][])
    n379 = Concatenate Strings(w57, "-Serial port output", ".txt" ("Suffix")) -> (w61:string)
    n380 = Build Array("Time /s" ("element"), "Id max /A" ("VAR2 Name"), "Id min /A" ("VAR2 Name"), "Absolute plunger position" ("VAR2 Name")) -> (w91:string[])
    n381 = Array To Spreadsheet String(array=w62, 3:"" ("format string")) -> (spreadsheet string=w67:string)  [unwired: 1 in]
    n382 = Transpose 2D Array(2D array=w84) -> (transposed array=w83:dbl[][])
    n383 = String To Path(string=w61) -> (path=w58:path)
    n384 = Concatenate Strings(w57, "Prefix (time data)", "Suffix (time data)") -> (w99:string)
    n385 = Array To Spreadsheet String(array=w91, 3:"" ("format string")) -> (spreadsheet string=w90:string)  [unwired: 1 in]
    n386 = Array To Spreadsheet String(array=w83, 3:"%e" ("format string")) -> (spreadsheet string=w89:string)  [unwired: 1 in]
    n387 = String To Path(string=w99) -> (path=w98:path)
    n388 = local write "Serial port data"(w67) -> ()
    n389 = Write to Text File(file (use dialog)=w58, text=w62, error in=w56) -> (refnum out=w63:refnum<file>, error out=w64:errorcluster)  [unwired: 1 in, 1 out]
    n390 = Build Array(w90, w89) -> (w88:string[])
    n391 = Close File(refnum=w63, error in=w64) -> (error out=w55:errorcluster)  [unwired: 1 out]
    n392 = Write to Text File(file (use dialog)=w98, text=w88, error in=w55) -> (refnum out=w100:refnum<file>, error out=w87:errorcluster)  [unwired: 1 in, 1 out]
    n393 = Close File(refnum=w100, error in=w87) -> (error out=w81:errorcluster)  [unwired: 1 out]
  }
  "error out" <- w9
